vi "EnFlo_Hub.vi"() -> ()   [LabVIEW 2013]
uses:
  Anemometry Sub Vis/Controls/Launch_controls/Open_Calib.ctl
  Anemometry Sub Vis/Controls/Launch_controls/Open_Meas.ctl
  Anemometry Sub Vis/Controls/Launch_controls/Open_Enter_Temp.ctl
  Anemometry Sub Vis/Controls/Launch_controls/Multi_Run_Prog.ctl
  Anemometry Sub Vis/Controls/Launch_controls/EnFlo_arm.ctl
  Anemometry Sub Vis/Controls/Launch_controls/Fast_FID_Valve.ctl
  Anemometry Sub Vis/Controls/Launch_controls/Disp_Setup.ctl
  Anemometry Sub Vis/Controls/Launch_controls/EnFlo_Tun_Setup.ctl
  Anemometry Sub Vis/Controls/Launch_controls/User_Metadata.ctl
  Anemometry Sub Vis/Controls/Launch_controls/Trav_3D_move.ctl
  Anemometry Sub Vis/Controls/Launch_controls/Trav_Space.ctl
  Anemometry Sub Vis/Controls/Launch_controls/Tunnel_speed.ctl
  Anemometry Sub Vis/Controls/Launch_controls/Client_source_control.ctl
  Anemometry Sub Vis/Controls/Launch_controls/Hydrosonic_Manual.ctl
  Anemometry Sub Vis/Controls/Launch_controls/Preference_Panel.ctl
  Anemometry Sub Vis/Controls/Launch_controls/Hot_wire_Calculator.ctl
  Anemometry Sub Vis/Controls/Launch_controls/RW_X_Parker_Config.ctl
  Anemometry Sub Vis/Controls/Launch_controls/LDA_Alignment.ctl
  Anemometry Sub Vis/Controls/Launch_controls/Named_Serial_Comms.ctl
  Anemometry Sub Vis/Controls/Launch_controls/BSA_data_rates.ctl
  Anemometry Sub Vis/Controls/Launch_controls/Serial_Setup.ctl
  Anemometry Sub Vis/Controls/Launch_controls/Post_Process_icon.ctl
  Anemometry Sub Vis/Controls/Launch_controls/Edit_Ascii_file.ctl
  Anemometry Sub Vis/Controls/Launch_controls/Edit_Raw_DF.ctl
  Anemometry Sub Vis/Controls/Launch_controls/Results_file_plotter.ctl
  Anemometry Sub Vis/Controls/Launch_controls/Serial_Port_Names.ctl
  Anemometry Sub Vis/Controls/Launch_controls/Paul.ctl
  Anemometry Sub Vis/Controls/Launch_controls/Tom.ctl
  Anemometry Sub Vis/Controls/Launch_controls/Scani_Valve.ctl
  Anemometry Sub Vis/Controls/Launch_controls/Edit_sever_Channel.ctl
  Anemometry Sub Vis/Controls/Launch_controls/Day_file_plotter.ctl
  Anemometry Sub Vis/Controls/Launch_controls/Plot_Sever_Data.ctl
  Anemometry Sub Vis/Controls/Launch_controls/Adam_Table.ctl
  Anemometry Sub Vis/Controls/Launch_controls/Active_Channel_Control.ctl
  Anemometry Sub Vis/Controls/Setup.ctl
  Anemometry Sub Vis/Controls/Post_Process.ctl
  Anemometry Sub Vis/Controls/Preference_Mode.ctl
  Anemometry Sub Vis/Gen Trav/Trav_mode.ctl
  Anemometry Sub Vis/Controls/User_Specific_mode.ctl
  Anemometry Sub Vis/File/Setup_Filetype.ctl
  Anemometry Sub Vis/Calibration/Calib_mode.ctl
  Anemometry Sub Vis/Controls/Server_Comms.ctl
  Anemometry Sub Vis/Controls/App_Global.ctl
  Anemometry Sub Vis/Globals/Dynamic_call_global.ph.vi
  Anemometry Sub Vis/Globals/Constants_global.vi
  Anemometry Sub Vis/Globals/Preference_global.vi
  Anemometry Sub Vis/Globals/Meas_global.vi
  <vilib>/Platform/browser.llb/Open URL in Default Browser (string).vi
  Anemometry Sub Vis/Globals/Trav_pos_global.vi
  Anemometry Sub Vis/Acquisition/PWA/PWAtasksGLOBAL.vi
  Anemometry Sub Vis/Utilities/Email_transfer_global.vi
panel:
  out "List of ADAM channels to view":string[](array[string])
  out "List of ADAM control channels":string[](array[string])
  out "Analogue Dev Name":string="Dev2"
  out "Numeric":i32
  out "Rig Name":string="EnFlo Tunnel"
  out "All Users":path=path "/System Folder/Preferences/LabVIEW (EnFlo specific)/Meas Setups"
  out "Dummy Measurement":bool
  in  "stop":bool
  in  "Tab Control":T1(tab)
  in  "Tunnel Speed Control":T2
  in  "Traverse Space":T3
  in  "Trav 3D Move":T4 caption="3D Traverse Move"
  in  "User Metadata":T5
  in  "Multi Run Prog":T6
  in  "Enter Temp_Press":T7
  in  "Measurement Prog":T8 caption="Measurement"
  in  "Calibration Prog":T9 caption="Calibration"
  in  "Scani Valve":T10
  in  "LDA Alignment":T11
  in  "Hydrosonic Control":T12
  in  "Fast FID Valve":T13
  in  "Source Control":T14
  in  "Gas Release Setup":T15
  in  "EnFlo Tunnel Setup":T16
  in  "Heater Setup":bool caption="Inlet heater File"
  in  "EnFlo Arm":T17
  in  "EnFlo Tun Display":bool
  in  "Rig_Control":cluster{"Ch Name":string, "Boolean":bool}[](array[cluster])
  in  "ADAM Channels Control":T18 caption="Change Active Channels"
  in  "ADAM Scan Table":T19 caption="Run ADAM Scan Table"
  in  "Edit Server Channel":T20
  in  "Plot Server Channels":T21 caption="Plot Server Data"
  in  "Day Files Plotter":T22 caption="Plot Data From File"
  out "Current Values":cluster{"Ch Name":string, "Numeric":dbl}[](array[cluster])
  in  "Post_Pro_Results_Hierarchy":bool
  in  "Results File Plotter":T23
  in  "Edit Raw Data Files":T24
  in  "Edit ASCII File":T25
  in  "Post Process Raw Data":T26
  in  "Top Level Traverse":bool
  in  "Show Manual Sync":bool
  in  "Sync to server now":bool
  in  "Port Names":T27
  in  "Serial Setup":T28
  in  "LDA Data Rate":T29
  in  "Named Serial Comms":T30
  in  "RW Trav Setup":T31
  in  "Hot Wire Calc":T32
  in  "Preference Panel":T33
  in  "Tom Lawton t.lawton@surrey.ac.uk":T34 caption="For hardware support"
  in  "Paul Hayden p.hayden@surrey.ac.uk":T35 caption="For software support"
  in  "Online Manual":bool
  out "VI Name":string
  out "Iterations":i32
  # "Or give us a call on Tel: 01483 689545"
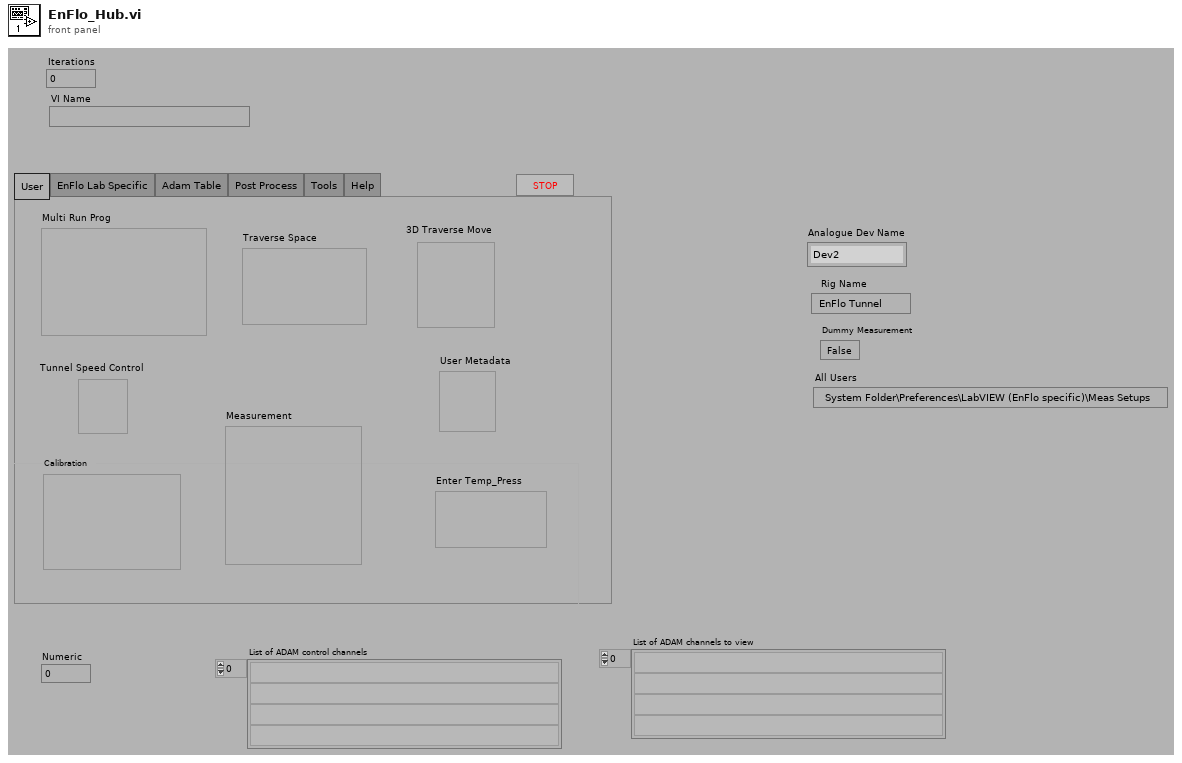
[diagram p1: front panel]
types:
  T1 = enum32{"User", "EnFlo Lab Specific", "Adam Table", "Post Process", "Tools", "Help"}
  T2 = typedef "Tunnel_speed.ctl" = bool
  T3 = typedef "Trav_Space.ctl" = bool
  T4 = typedef "Trav_3D_move.ctl" = bool
  T5 = typedef "User_Metadata.ctl" = bool
  T6 = typedef "Multi_Run_Prog.ctl" = bool
  T7 = typedef "Open_Enter_Temp.ctl" = bool
  T8 = typedef "Open_Meas.ctl" = bool
  T9 = typedef "Open_Calib.ctl" = bool
  T10 = typedef "Scani_Valve.ctl" = bool
  T11 = typedef "LDA_Alignment.ctl" = bool
  T12 = typedef "Hydrosonic_Manual.ctl" = bool
  T13 = typedef "Fast_FID_Valve.ctl" = bool
  T14 = typedef "Client_source_control.ctl" = bool
  T15 = typedef "Disp_Setup.ctl" = bool
  T16 = typedef "EnFlo_Tun_Setup.ctl" = bool
  T17 = typedef "EnFlo_arm.ctl" = bool
  T18 = typedef "Active_Channel_Control.ctl" = bool
  T19 = typedef "Adam_Table.ctl" = bool
  T20 = typedef "Edit_sever_Channel.ctl" = bool
  T21 = typedef "Plot_Sever_Data.ctl" = bool
  T22 = typedef "Day_file_plotter.ctl" = bool
  T23 = typedef "Results_file_plotter.ctl" = bool
  T24 = typedef "Edit_Raw_DF.ctl" = bool
  T25 = typedef "Edit_Ascii_file.ctl" = bool
  T26 = typedef "Post_Process_icon.ctl" = bool
  T27 = typedef "Serial_Port_Names.ctl" = bool
  T28 = typedef "Serial_Setup.ctl" = bool
  T29 = typedef "BSA_data_rates.ctl" = bool
  T30 = typedef "Named_Serial_Comms.ctl" = bool
  T31 = typedef "RW_X_Parker_Config.ctl" = bool
  T32 = typedef "Hot_wire_Calculator.ctl" = bool
  T33 = typedef "Preference_Panel.ctl" = bool
  T34 = typedef "Tom.ctl" = bool
  T35 = typedef "Paul.ctl" = bool
  T36 = enum32{"invalid app kind", "Development System", "Run Time System", "Student Edition", "Embedded LabVIEW", "Evaluation", "Custom"}
  T37 = typedef "Post_Process.ctl" = enum16{"Take New Data", "Post Process Raw Data File"}
  T38 = typedef "Setup.ctl" = enum16{"Run Program", "Show Setup", "Save Current Setup", "Setup Front Panel"}
  T39 = enum16{"Get Channel Names", "Get Current Value", "Update Channel Value", "Update Channel Description"}
  T40 = enum32{"Invalid", "Standard", "Closed", "Hidden", "Minimized", "Maximized"}
  T41 = typedef "Preference_Mode.ctl" = enum16{"Load Preferences from file", "Save Preferences to file", "Load, Edit then Save"}
  T42 = typedef "User_Specific_mode.ctl" = enum16{"Check VI only", "Run VI"}
  T43 = typedef "Trav_mode.ctl" = enum16{"Move traverse", "Read traverse position", "Teach Position"}
  T44 = typedef "Setup_Filetype.ctl" = enum16{"Measurement Setups", "Calibration Setups", "General", "Results File Plotter Setups", "Speed Calib Tweaks"}
  T45 = enum16{"Load Command File", "Save Command File", "Check Multi Run Prog", "Check Multi Run Prog With Live Moves", "Run Multi Run Prog"}
  T46 = typedef "Calib_mode.ctl" = enum16{"Show Setup", "Take a New Calibration Point", "Refit Curve", "Setup Front Panel"}
  T47 = typedef "Tunnel_Coordinates.ctl" = enum16{"Work in Tunnel Coordinates", "Work in Model Coordinates"}
  T48 = typedef "App_Global.ctl" = enum16{"Read Global", "Write to Global", "Initialise Array"}
  T49 = typedef "App_Ref_Cluster.ctl" = cluster{"Server IP & Port No":string, "Application reference":refnum<vi>}
  T50 = typedef "Server_Comms.ctl" = enum16{"Server Link Healthy", "Do Not Link To Server"}
  T51 = typedef "Ch_description_ADAM.ctl" = cluster{"Ch Name":string, "Type":T52, "Function":T53, "Ch State":T54, "Calibration type":T55, "A":dbl, "B":dbl, "C":dbl, "D":dbl, "Comments":string, "Address":T56, "String":string, "Duty":u16}
  T52 = typedef "Module_type_ADAM.ctl" = string
  T53 = typedef "Function_ADAM.ctl" = enum16{"Analogue Input", "Digital Input", "Event counter", "Event rate", "Analogue Output", "Digital Output", "Relay Output"}
  T54 = typedef "Channel_State.ctl" = enum16{"On", "Off", "Always On", "Always Off"}
  T55 = typedef "Calib_type_ADAM.ctl" = enum16{"Raw", "Bx + A", "Cx^2 + Bx + A", "Dx^3 + Cx^2 + Bx + A", "In Band", "Hi-Tec Q", "Hi-Tec M_dot", "Text"}
  T56 = typedef "Address.ctl" = cluster{"Main":i32, "Ch.":i32, "Sub":i32, "Port Name":string}
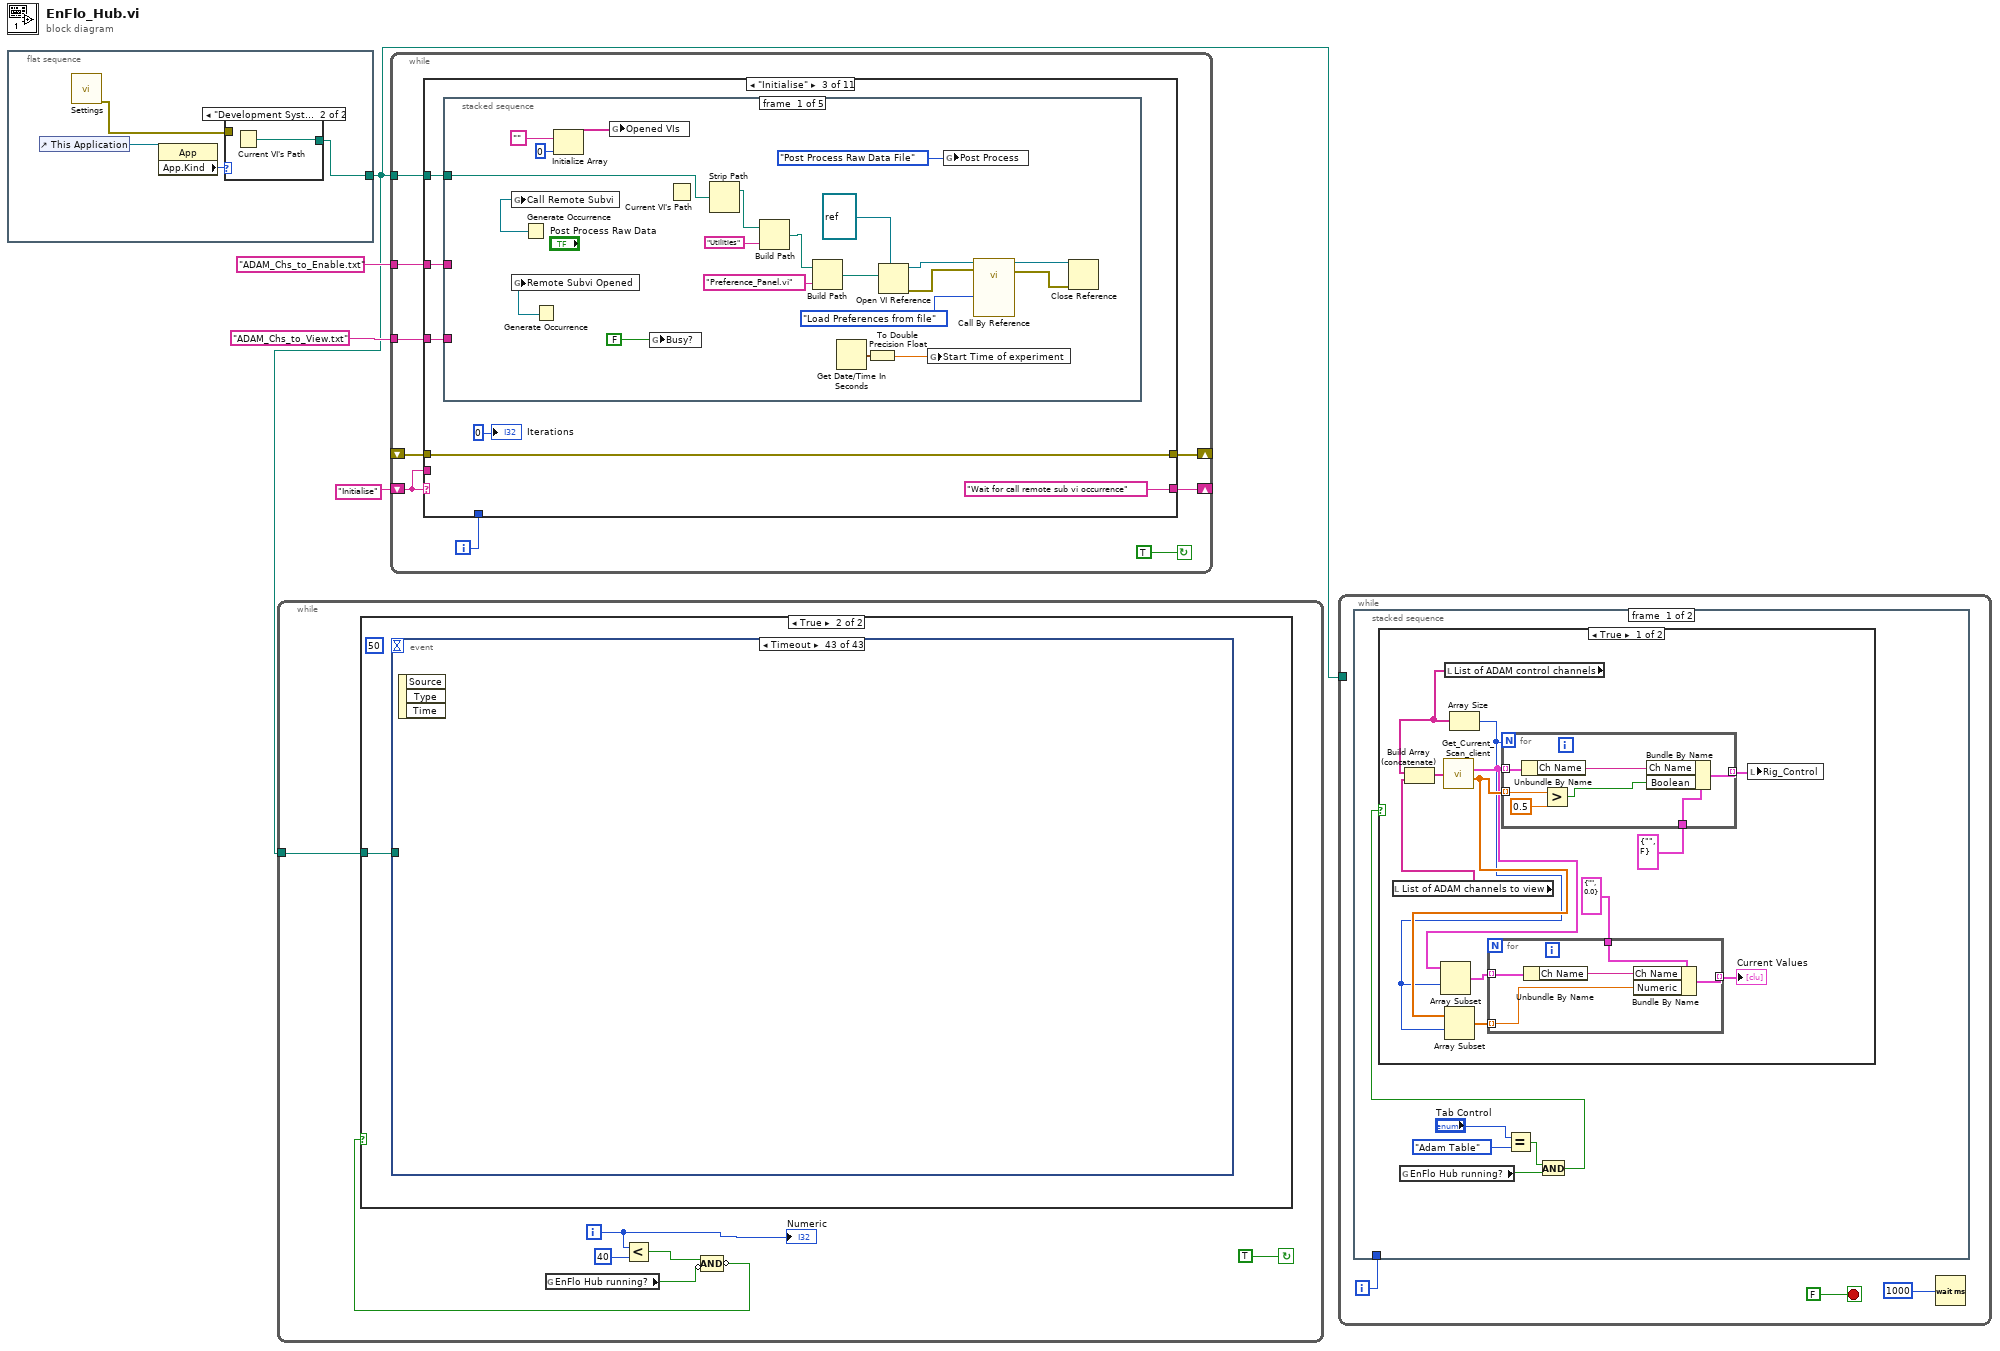
[diagram p0: block diagram]
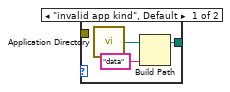
[diagram p2: hidden frame]
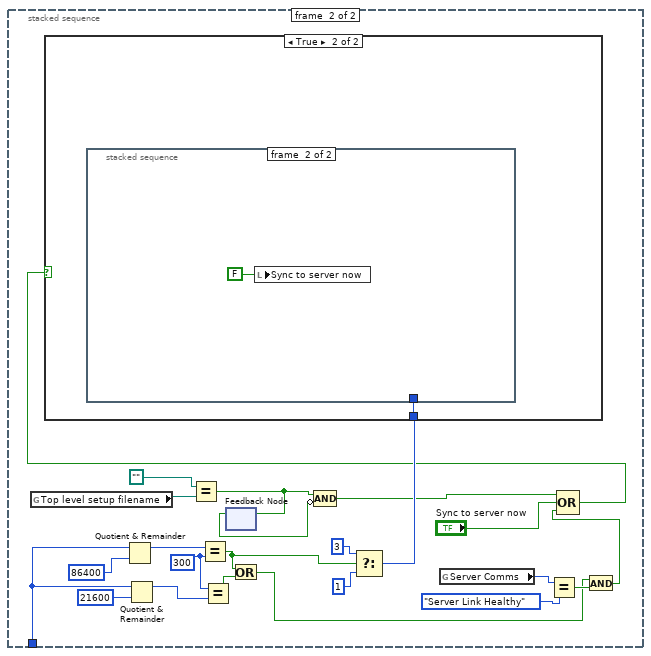
[diagram p4: hidden frame]
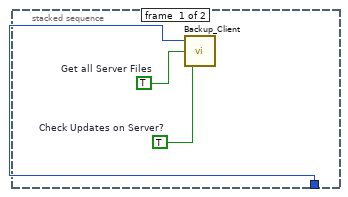
[diagram p6: hidden frame]
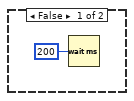
[diagram p7: hidden frame]
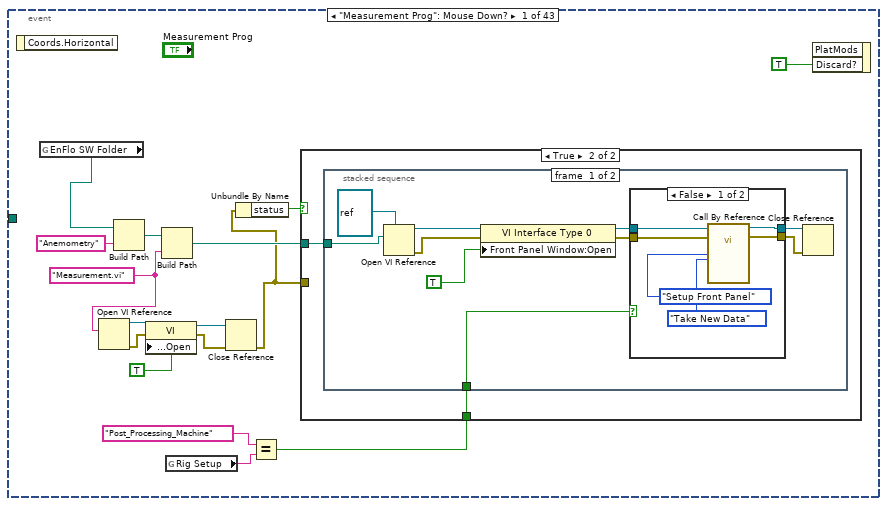
[diagram p8: hidden frame]
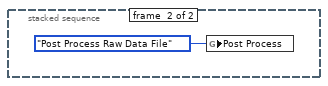
[diagram p11: hidden frame]
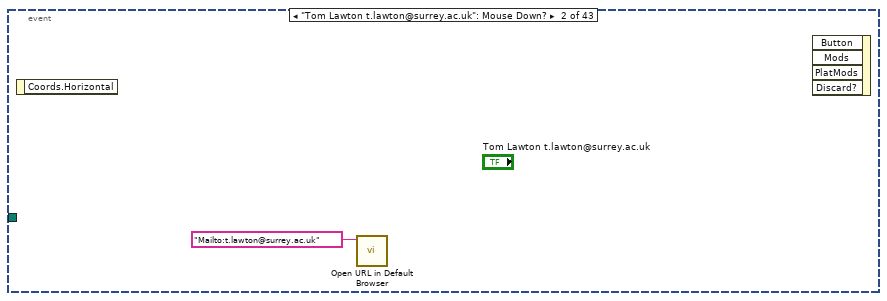
[diagram p12: hidden frame]
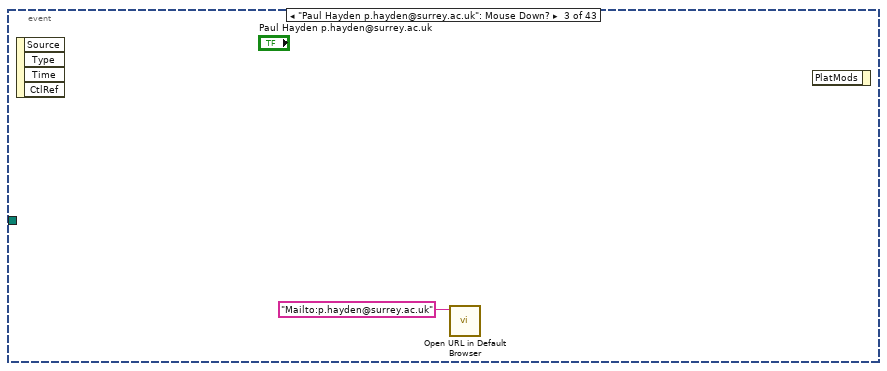
[diagram p13: hidden frame]
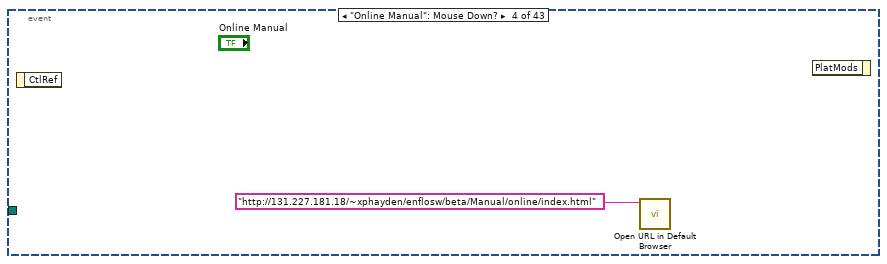
[diagram p14: hidden frame]
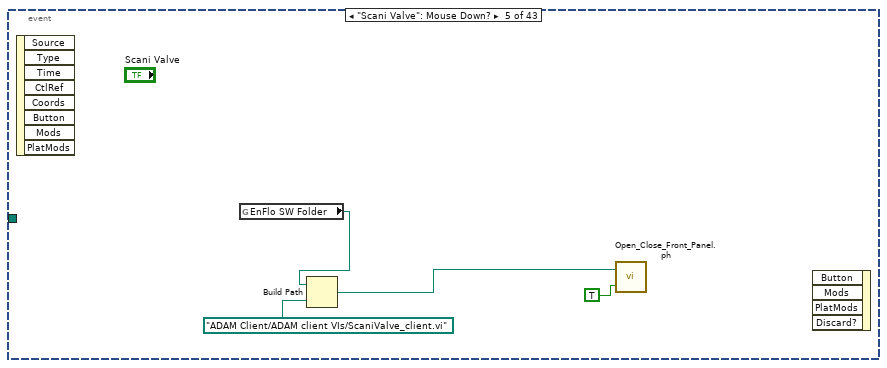
[diagram p15: hidden frame]
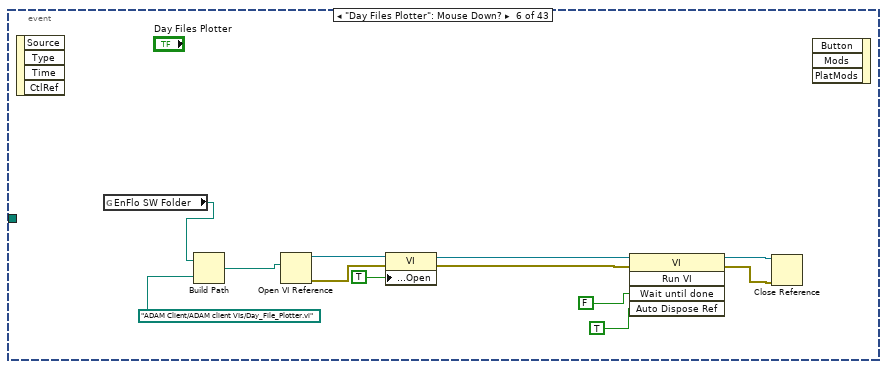
[diagram p16: hidden frame]
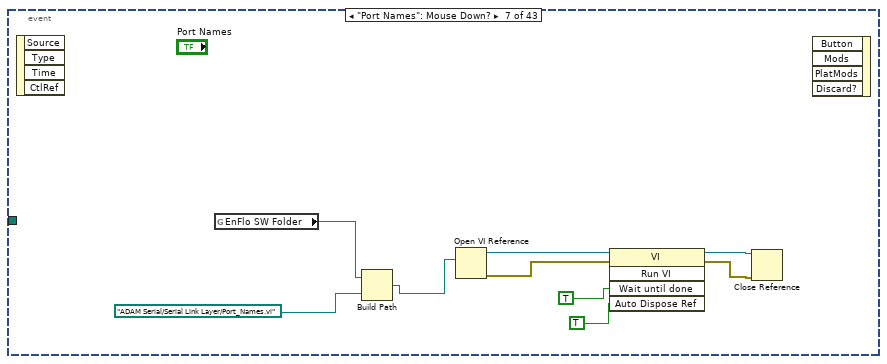
[diagram p17: hidden frame]
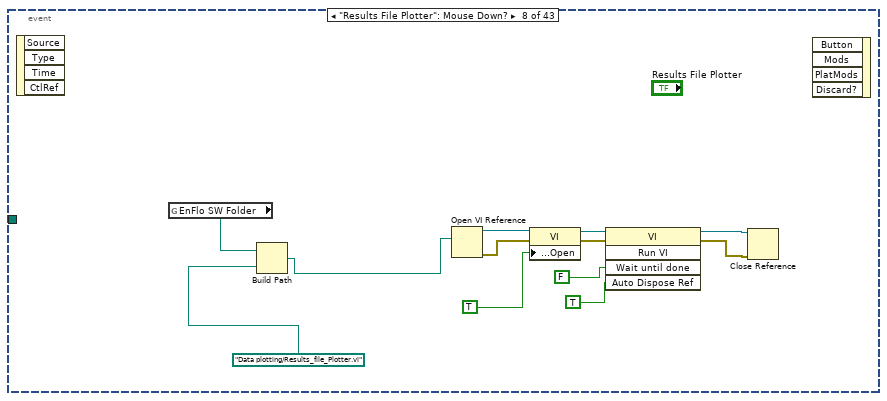
[diagram p18: hidden frame]
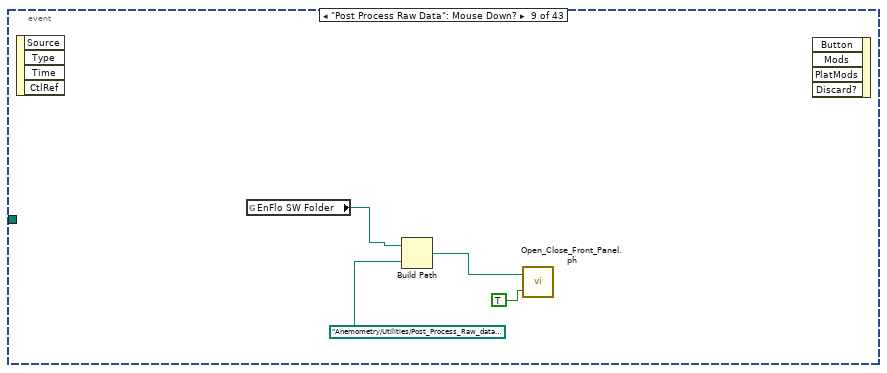
[diagram p19: hidden frame]
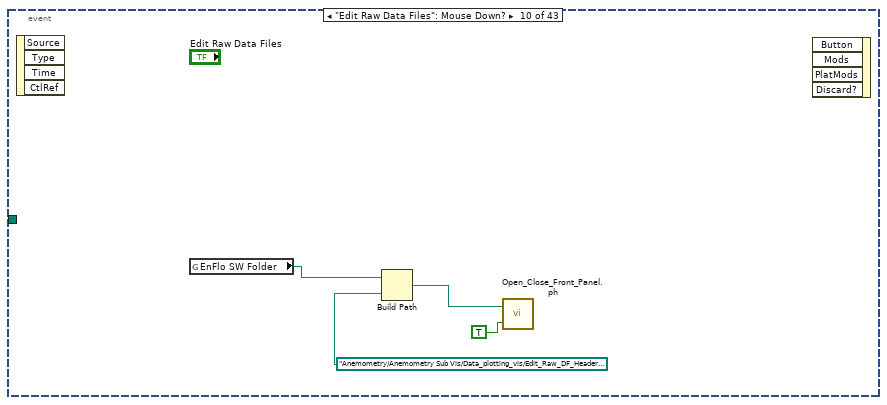
[diagram p20: hidden frame]
diagram:
  n1 = flat-sequence {
    tunnel: [w8] -> w1
    frame #0 {
      n2 = control-ref of="This Application"() -> (w6:refnum<vi>)
      n3 = call "Settings.vi"() -> ("error out"=w5:errorcluster)  [unwired: 11 in]
      n4 = property class="App"(reference=w6) -> ("App.Kind"=w7:T36)  [unwired: 1 in, 2 out]
      n5 = case shown="\"Development System\"" w7 {
        tunnel: [w11 w12] -> w8
        tunnel: w5 -> [_ _]
        frame "invalid app kind", Default {
          n6 = call <vilib>:"Application Directory.vi"() -> ("Application Directory"=w9:path)
          n7 = Build Path(base path=w9, name or relative path="data") -> (appended path=w11:path)
        }
        frame "Development System" {
          n8 = Current VI's Path() -> (path=w12:path)
        }
      }
    }
  }
  n9 = while {
    tunnel: w1 -> [w13]
    i -> [w18]
    stop <- TRUE continue-if-true
    n10 = global read "Dynamic_call_global.ph.vi" "EnFlo Hub running?"() -> (w16:bool)
    n11 = Less?(x=w18, y=40) -> (x < y?=w15:bool)
    n12 = Compound Arithmetic op=AND(w15, invert w16) -> (invert w14:bool)
    n13 = case shown="True" w14 {
      tunnel: w13 -> [_ w21]
      frame False {
        n14 = Wait (ms)(milliseconds to wait=u32 200) -> ()  [unwired: 1 out]
      }
      frame True {
        (unwired) 50
        n15 = event shown="[42] Timeout" {
          selector: _ -> [_ _ _ _ _ _ _ _ _ _ _ _ _ _ _ _ _ _ _ _ _ _ _ _ _ _ _ _ _ _ _ _ _ _ _ _ _ _ _ _ _ _ _]
          dyn-events: _ -> [_ _ _ _ _ _ _ _ _ _ _ _ _ _ _ _ _ _ _ _ _ _ _ _ _ _ _ _ _ _ _ _ _ _ _ _ _ _ _ _ _ _ _]
          timeout: _ -> [_ _ _ _ _ _ _ _ _ _ _ _ _ _ _ _ _ _ _ _ _ _ _ _ _ _ _ _ _ _ _ _ _ _ _ _ _ _ _ _ _ _ _]
          tunnel: w21 -> [_ _ _ _ _ _ _ _ _ _ _ _ _ _ _ _ _ _ _ _ _ _ _ _ _ _ _ _ _ _ _ _ _ _ _ _ _ _ _ _ _ _ _]
          event "Measurement Prog": Mouse Down? {
            w30 = "Measurement.vi" ("name or relative path")
            n16 = event-data() -> ()  [unwired: 2 out]
            n17 = global read "Constants_global.vi" "EnFlo SW Folder"() -> (w33:path)
            n18 = Open VI Reference(vi path=w30) -> (vi reference=w29:refnum<vi>, error out=w28:errorcluster)  [unwired: 1 in, 4 out]
            n19 = Build Path(base path=w33, name or relative path="Anemometry") -> (appended path=w36:path)
            n20 = property class="VI"(reference=w29, error in=w28, "Front Panel Window:Open"=TRUE) -> (reference out=w26:refnum<vi>, error out=w27:errorcluster)
            n21 = Build Path(base path=w36, name or relative path=w30) -> (appended path=w34:path)
            n22 = global read "Preference_global.vi" "Rig Setup"() -> (w24:string)
            n23 = Close Reference(reference=w26, error in (no error)=w27) -> (error out=w25:errorcluster)
            n24 = Unbundle By Name(w25) -> ("status"=w35:bool)
            n25 = Equal?(x="Post_Processing_Machine" ("Rig Setup"), y=w24) -> (x = y?=w22:bool)
            n26 = case shown="True" w35 {
              tunnel: w34 -> [_ w39]
              tunnel: w25 -> [_ _]
              tunnel: w22 -> [_ w38]
              frame False {
              }
              frame True {
                n27 = stacked-sequence {
                  tunnel: w39 -> [w49 _]
                  tunnel: w38 -> [w40 _]
                  frame #0 {
                    n28 = Open VI Reference(type specifier VI Refnum (for type only)=refnum<vi> refnum, vi path=w49) -> (vi reference=w47:refnum<vi>, error out=w46:errorcluster)  [unwired: 1 in, 3 out]
                    n29 = property class="VI Interface Type 0"(reference=w47, error in=w46, "Front Panel Window:Open"=TRUE) -> (reference out=w42:refnum<vi>, error out=w41:errorcluster)
                    n30 = case shown="False" w40 {
                      tunnel: [w55 w57] -> w45
                      tunnel: [w54 w56] -> w44
                      tunnel: w42 -> [w53 w57]
                      tunnel: w41 -> [w52 w56]
                      frame False {
                        n31 = call-by-ref "?"(reference=w53, error in=w52, "setup"=Setup."Setup Front Panel", "Post Process"=Post_Process."Take New Data") -> (reference out=w55:refnum<vi>, error out=w54:errorcluster)  [unwired: 16 in, 2 out]
                      }
                      frame True {
                      }
                    }
                    n32 = Close Reference(reference=w45, error in (no error)=w44) -> ()  [unwired: 1 out]
                  }
                  frame #1 {
                    n33 = global write "Meas_global.vi" "Post Process"(Post_Process."Post Process Raw Data File" ("Post Process")) -> ()
                  }
                }
              }
            }
            n34 = event-data("Discard?"=TRUE) -> ()  [unwired: 1 in, 2 out]
          }
          event "Tom Lawton t.lawton@surrey.ac.uk": Mouse Down? {
            n35 = event-data() -> ()  [unwired: 2 out]
            n36 = call-poly <vilib>:"Open URL in Default Browser.vi"("URL"="Mailto:t.lawton@surrey.ac.uk") -> ()  [unwired: 1 in, 6 out]
            n37 = event-data() -> ()  [unwired: 1 in, 5 out]
          }
          event "Paul Hayden p.hayden@surrey.ac.uk": Mouse Down? {
            n38 = event-data() -> ()  [unwired: 5 out]
            n39 = call-poly <vilib>:"Open URL in Default Browser.vi"("URL"="Mailto:p.hayden@surrey.ac.uk") -> ()  [unwired: 1 in, 6 out]
            n40 = event-data() -> ()  [unwired: 1 in, 2 out]
          }
          event "Online Manual": Mouse Down? {
            n41 = event-data() -> ()  [unwired: 2 out]
            n42 = call-poly <vilib>:"Open URL in Default Browser.vi"("URL"="http://131.227.181.18/~xphayden/enflosw/beta/Manual/online/index.html") -> ()  [unwired: 1 in, 6 out]
            n43 = event-data() -> ()  [unwired: 1 in, 2 out]
          }
          event "Scani Valve": Mouse Down? {
            n44 = event-data() -> ()  [unwired: 9 out]
            n45 = global read "Constants_global.vi" "EnFlo SW Folder"() -> (w62:path)
            n46 = Build Path(base path=w62, name or relative path=path "ADAM Client/ADAM client VIs/ScaniValve_client.vi") -> (appended path=w65:path)
            n47 = call "Open_Close_Front_Panel.ph.vi"("Front Panel Window:Open"=TRUE, "VI path"=w65) -> ()  [unwired: 2 out]
            n48 = event-data() -> ()  [unwired: 1 in, 5 out]
          }
          event "Day Files Plotter": Mouse Down? {
            n49 = event-data() -> ()  [unwired: 5 out]
            n50 = global read "Constants_global.vi" "EnFlo SW Folder"() -> (w66:path)
            n51 = Build Path(base path=w66, name or relative path=path "ADAM Client/ADAM client VIs/Day_File_Plotter.vi") -> (appended path=w72:path)
            n52 = Open VI Reference(vi path=w72) -> (vi reference=w73:refnum<vi>, error out=w75:errorcluster)  [unwired: 2 in, 3 out]
            n53 = property class="VI"(reference=w73, error in=w75, "Front Panel Window:Open"=TRUE) -> (reference out=w77:refnum<vi>, error out=w76:errorcluster)
            n54 = invoke class="VI" method="Run VI"(reference=w77, error in=w76, "Wait until done"=FALSE, "Auto Dispose Ref"=TRUE) -> (reference out=w68:refnum<vi>, error out=w69:errorcluster)  [unwired: 1 in, 3 out]
            n55 = Close Reference(reference=w68, error in (no error)=w69) -> ()  [unwired: 1 out]
            n56 = event-data() -> ()  [unwired: 1 in, 4 out]
          }
          event "Port Names": Mouse Down? {
            n57 = event-data() -> ()  [unwired: 5 out]
            n58 = global read "Constants_global.vi" "EnFlo SW Folder"() -> (w78:path)
            n59 = Build Path(base path=w78, name or relative path=path "ADAM Serial/Serial Link Layer/Port_Names.vi") -> (appended path=w80:path)
            n60 = Open VI Reference(vi path=w80) -> (vi reference=w85:refnum<vi>, error out=w86:errorcluster)  [unwired: 1 in, 4 out]
            n61 = invoke class="VI" method="Run VI"(reference=w85, error in=w86, "Wait until done"=TRUE, "Auto Dispose Ref"=TRUE) -> (reference out=w81:refnum<vi>, error out=w82:errorcluster)  [unwired: 1 in, 3 out]
            n62 = Close Reference(reference=w81, error in (no error)=w82) -> ()  [unwired: 1 out]
            n63 = event-data() -> ()  [unwired: 1 in, 5 out]
          }
          event "Results File Plotter": Mouse Down? {
            n64 = event-data() -> ()  [unwired: 5 out]
            n65 = global read "Constants_global.vi" "EnFlo SW Folder"() -> (w87:path)
            n66 = Build Path(base path=w87, name or relative path=path "Data plotting/Results_file_Plotter.vi") -> (appended path=w90:path)
            n67 = Open VI Reference(vi path=w90) -> (vi reference=w92:refnum<vi>, error out=w89:errorcluster)  [unwired: 1 in, 4 out]
            n68 = property class="VI"(reference=w92, error in=w89, "Front Panel Window:Open"=TRUE) -> (reference out=w93:refnum<vi>, error out=w94:errorcluster)
            n69 = invoke class="VI" method="Run VI"(reference=w93, error in=w94, "Wait until done"=FALSE, "Auto Dispose Ref"=TRUE) -> (reference out=w95:refnum<vi>, error out=w96:errorcluster)  [unwired: 1 in, 3 out]
            n70 = Close Reference(reference=w95, error in (no error)=w96) -> ()  [unwired: 1 out]
            n71 = event-data() -> ()  [unwired: 1 in, 5 out]
          }
          event "Post Process Raw Data": Mouse Down? {
            n72 = event-data() -> ()  [unwired: 5 out]
            n73 = global read "Constants_global.vi" "EnFlo SW Folder"() -> (w99:path)
            n74 = Build Path(base path=w99, name or relative path=path "Anemometry/Utilities/Post_Process_Raw_data.vi") -> (appended path=w101:path)
            n75 = call "Open_Close_Front_Panel.ph.vi"("Front Panel Window:Open"=TRUE, "VI path"=w101) -> ()  [unwired: 2 out]
            n76 = event-data() -> ()  [unwired: 1 in, 5 out]
          }
          event "Edit Raw Data Files": Mouse Down? {
            n77 = event-data() -> ()  [unwired: 5 out]
            n78 = global read "Constants_global.vi" "EnFlo SW Folder"() -> (w103:path)
            n79 = Build Path(base path=w103, name or relative path=path "Anemometry/Anemometry Sub Vis/Data_plotting_vis/Edit_Raw_DF_Header.vi") -> (appended path=w105:path)
            n80 = call "Open_Close_Front_Panel.ph.vi"("Front Panel Window:Open"=TRUE, "VI path"=w105) -> ()  [unwired: 2 out]
            n81 = event-data() -> ()  [unwired: 1 in, 5 out]
          }
          event "Serial Setup": Mouse Down? {
            n82 = event-data() -> ()  [unwired: 5 out]
            n83 = global read "Constants_global.vi" "EnFlo SW Folder"() -> (w107:path)
            n84 = Build Path(base path=w107, name or relative path=path "ADAM Serial/Serial Link Layer/Serial_Setup.vi") -> (appended path=w109:path)
            n85 = Open VI Reference(vi path=w109) -> (vi reference=w114:refnum<vi>, error out=w115:errorcluster)  [unwired: 1 in, 4 out]
            n86 = invoke class="VI" method="Run VI"(reference=w114, error in=w115, "Wait until done"=TRUE, "Auto Dispose Ref"=TRUE) -> (reference out=w110:refnum<vi>, error out=w111:errorcluster)  [unwired: 1 in, 3 out]
            n87 = Close Reference(reference=w110, error in (no error)=w111) -> ()  [unwired: 1 out]
            n88 = event-data() -> ()  [unwired: 1 in, 2 out]
          }
          event "Named Serial Comms": Mouse Down? {
            n89 = event-data() -> ()  [unwired: 5 out]
            n90 = global read "Constants_global.vi" "EnFlo SW Folder"() -> (w117:path)
            n91 = Build Path(base path=w117, name or relative path=path "ADAM Serial/Serial Link Layer/Named_Serial_Comms.vi") -> (appended path=w119:path)
            n92 = call "Open_Close_Front_Panel.ph.vi"("Front Panel Window:Open"=TRUE, "VI path"=w119) -> ()  [unwired: 2 out]
            n93 = event-data() -> ()  [unwired: 1 in, 5 out]
          }
          event "LDA Data Rate": Mouse Down? {
            n94 = event-data() -> ()  [unwired: 5 out]
            n95 = global read "Constants_global.vi" "EnFlo SW Folder"() -> (w120:path)
            n96 = Build Path(base path=w120, name or relative path=path "Anemometry/Anemometry Sub Vis/LDA/LDA_data_rate.vi") -> (appended path=w122:path)
            n97 = call "Open_Close_Front_Panel.ph.vi"("Front Panel Window:Open"=TRUE, "VI path"=w122) -> ()  [unwired: 2 out]
            n98 = event-data() -> ()  [unwired: 1 in, 2 out]
          }
          event "ADAM Channels Control": Mouse Down? {
            n99 = event-data() -> ()  [unwired: 5 out]
            n100 = global read "Constants_global.vi" "EnFlo SW Folder"() -> (w134:path)
            n101 = Build Path(base path=w134, name or relative path=path "ADAM Client/ADAM client VIs/Control_Channel_Status.vi") -> (appended path=w124:path)
            n102 = Open VI Reference(vi path=w124) -> (vi reference=w127:refnum<vi>, error out=w125:errorcluster)  [unwired: 1 in, 4 out]
            n103 = property class="VI"(reference=w127, error in=w125, "Front Panel Window:Open"=TRUE) -> (reference out=w128:refnum<vi>, error out=w129:errorcluster)
            n104 = invoke class="VI" method="Run VI"(reference=w128, error in=w129, "Wait until done"=FALSE, "Auto Dispose Ref"=TRUE) -> (reference out=w130:refnum<vi>, error out=w131:errorcluster)  [unwired: 1 in, 3 out]
            n105 = Close Reference(reference=w130, error in (no error)=w131) -> ()  [unwired: 1 out]
            n106 = event-data() -> ()  [unwired: 1 in, 2 out]
          }
          event "LDA Alignment": Mouse Down? {
            n107 = event-data() -> ()  [unwired: 5 out]
            n108 = global read "Constants_global.vi" "EnFlo SW Folder"() -> (w136:path)
            n109 = Build Path(base path=w136, name or relative path=path "Anemometry/Utilities/LDA_Beam_Alignment.vi") -> (appended path=w138:path)
            n110 = call "Open_Close_Front_Panel.ph.vi"("Front Panel Window:Open"=TRUE, "VI path"=w138) -> ()  [unwired: 2 out]
            n111 = event-data() -> ()  [unwired: 1 in, 5 out]
          }
          event "Enter Temp_Press": Mouse Down? {
            w141 = FALSE  # Wait until done
            n112 = event-data() -> ()  [unwired: 5 out]
            n113 = call "Run_Enter_Temp.vi"("Wait until done"=w141) -> ()  [unwired: 1 out]
            n114 = event-data("Discard?"=TRUE) -> ()  [unwired: 1 in, 4 out]
          }
          event "Edit ASCII File": Mouse Down? {
            n115 = event-data() -> ()  [unwired: 5 out]
            n116 = global read "Constants_global.vi" "EnFlo SW Folder"() -> (w142:path)
            n117 = Build Path(base path=w142, name or relative path=path "Anemometry/Utilities/Edit_ASCI_file.vi") -> (appended path=w145:path)
            n118 = call "Open_Close_Front_Panel.ph.vi"("Front Panel Window:Open"=TRUE, "VI path"=w145) -> ()  [unwired: 2 out]
            n119 = event-data() -> ()  [unwired: 1 in, 5 out]
          }
          event "Heater Setup": Mouse Down? {
            n120 = event-data() -> ()  [unwired: 5 out]
            n121 = global read "Constants_global.vi" "EnFlo SW Folder"() -> (w146:path)
            n122 = Build Path(base path=w146, name or relative path=path "Anemometry/Utilities/Create_Heater_Setpoints_File.vi") -> (appended path=w149:path)
            n123 = call "Open_Close_Front_Panel.ph.vi"("Front Panel Window:Open"=TRUE, "VI path"=w149) -> ()  [unwired: 2 out]
            n124 = event-data() -> ()  [unwired: 1 in, 5 out]
          }
          event "Source Control": Mouse Down? {
            n125 = event-data() -> ()  [unwired: 5 out]
            n126 = global read "Constants_global.vi" "EnFlo SW Folder"() -> (w150:path)
            n127 = Build Path(base path=w150, name or relative path=path "ADAM Client/Sub VIs/Gas_Release_Control.vi") -> (appended path=w153:path)
            n128 = call "Open_Close_Front_Panel.ph.vi"("Front Panel Window:Open"=TRUE, "VI path"=w153) -> ()  [unwired: 2 out]
            n129 = event-data() -> ()  [unwired: 1 in, 5 out]
          }
          event "Edit Server Channel": Mouse Down? {
            n130 = event-data() -> ()  [unwired: 5 out]
            n131 = global read "Constants_global.vi" "EnFlo SW Folder"() -> (w154:path)
            n132 = Build Path(base path=w154, name or relative path=path "ADAM Client/ADAM client VIs/Edit_Server_Channel.vi") -> (appended path=w164:path)
            n133 = Open VI Reference(type specifier VI Refnum (for type only)=refnum<vi> refnum, vi path=w164) -> (vi reference=w157:refnum<vi>, error out=w158:errorcluster)  [unwired: 1 in, 3 out]
            n134 = property class="VI Interface Type 1"(reference=w157, error in=w158, "Front Panel Window:Open"=TRUE) -> (reference out=w160:refnum<vi>, error out=w161:errorcluster)
            n135 = call-by-ref "?"(reference=w160, error in=w161, "Mode"=T39."Get Channel Names") -> (reference out=w162:refnum<vi>, error out=w163:errorcluster)  [unwired: 5 in]
            n136 = Close Reference(reference=w162, error in (no error)=w163) -> ()  [unwired: 1 out]
            n137 = event-data() -> ()  [unwired: 1 in, 5 out]
          }
          event "EnFlo Tun Display": Mouse Down? {
            n138 = event-data() -> ()  [unwired: 9 out]
            n139 = global read "Constants_global.vi" "EnFlo SW Folder"() -> (w177:path)
            n140 = Build Path(base path=w177, name or relative path=path "Anemometry/Utilities/EnFlo_Tunnel_Display.vi") -> (appended path=w172:path)
            n141 = Open VI Reference(vi path=w172) -> (vi reference=w171:refnum<vi>, error out=w170:errorcluster)  [unwired: 5 in]
            n142 = invoke class="VI" method="FP.Open"(reference=w171, error in=w170, "Activate"=TRUE ("Activate?"), "State"=T40."Standard") -> (reference out=w169:refnum<vi>, error out=w168:errorcluster)  [unwired: 1 in, 3 out]
            n143 = invoke class="VI" method="Run VI"(reference=w169, error in=w168, "Wait until done"=FALSE ("Wait Until Done"), "Auto Dispose Ref"=FALSE ("Wait until done")) -> (reference out=w173:refnum<vi>, error out=w174:errorcluster)  [unwired: 1 in, 3 out]
            n144 = Close Reference(reference=w173, error in (no error)=w174) -> ()  [unwired: 1 out]
            n145 = event-data() -> ()  [unwired: 5 in, 1 out]
          }
          event "Tunnel Speed Control": Mouse Down? {
            n146 = event-data() -> ()  [unwired: 5 out]
            n147 = global read "Constants_global.vi" "EnFlo SW Folder"() -> (w179:path)
            n148 = Build Path(base path=w179, name or relative path=path "ADAM Client/ADAM client VIs/Set_Tunnel_Speed.vi") -> (appended path=w182:path)
            n149 = call "Open_Close_Front_Panel.ph.vi"("Front Panel Window:Open"=TRUE, "VI path"=w182) -> ()  [unwired: 2 out]
            n150 = event-data() -> ()  [unwired: 1 in, 5 out]
          }
          event "Plot Server Channels": Mouse Down? {
            n151 = event-data() -> ()  [unwired: 5 out]
            n152 = global read "Constants_global.vi" "EnFlo SW Folder"() -> (w183:path)
            n153 = Build Path(base path=w183, name or relative path=path "ADAM Client/ADAM client VIs/Plot_Server_Data.vi") -> (appended path=w186:path)
            n154 = Open VI Reference(vi path=w186) -> (vi reference=w188:refnum<vi>, error out=w185:errorcluster)  [unwired: 1 in, 4 out]
            n155 = property class="VI"(reference=w188, error in=w185, "Front Panel Window:Open"=TRUE) -> (reference out=w189:refnum<vi>, error out=w190:errorcluster)
            n156 = invoke class="VI" method="Run VI"(reference=w189, error in=w190, "Wait until done"=FALSE, "Auto Dispose Ref"=TRUE) -> (reference out=w191:refnum<vi>, error out=w192:errorcluster)  [unwired: 1 in, 3 out]
            n157 = Close Reference(reference=w191, error in (no error)=w192) -> ()  [unwired: 1 out]
            n158 = event-data() -> ()  [unwired: 1 in, 5 out]
          }
          event "ADAM Scan Table": Mouse Down? {
            n159 = event-data() -> ()  [unwired: 5 out]
            n160 = Two Button Dialog(message="Are you sure that you want to Run the ADAM Scan table on this machine?", 1:"Run" ("F button name (\"Cancel\")"), 2:"Cancel" ("T button name (\"OK\")")) -> (T button?=w196:bool)
            n161 = case shown="False" w196 {
              frame False {
                n162 = global read "Constants_global.vi" "EnFlo SW Folder"() -> (w199:path)
                n163 = Build Path(base path=w199, name or relative path=path "ADAM Server/ADAM_scan_table.vi") -> (appended path=w202:path)
                n164 = Open VI Reference(vi path=w202) -> (vi reference=w204:refnum<vi>, error out=w201:errorcluster)  [unwired: 1 in, 4 out]
                n165 = property class="VI"(reference=w204, error in=w201, "Front Panel Window:Open"=TRUE) -> (reference out=w205:refnum<vi>, error out=w206:errorcluster)
                n166 = invoke class="VI" method="Run VI"(reference=w205, error in=w206, "Wait until done"=FALSE, "Auto Dispose Ref"=TRUE) -> (reference out=w207:refnum<vi>, error out=w208:errorcluster)  [unwired: 1 in, 3 out]
                n167 = Close Reference(reference=w207, error in (no error)=w208) -> ()  [unwired: 1 out]
              }
              frame True {
              }
            }
            n168 = event-data() -> ()  [unwired: 1 in, 2 out]
          }
          event "RW Trav Setup": Mouse Down? {
            n169 = event-data() -> ()  [unwired: 5 out]
            n170 = global read "Constants_global.vi" "EnFlo SW Folder"() -> (w213:path)
            n171 = Build Path(base path=w213, name or relative path=path "ADAM Serial/Instrument drivers/Traverses/~subVIs/Read_Write_Trav_Config.vi") -> (appended path=w214:path)
            n172 = Build Path(base path=w213, name or relative path=path "ADAM Serial/Instrument drivers/Traverses/~subVIs/DriveConfigGlobal.vi") -> (appended path=w215:path)
            n173 = flat-sequence {
              tunnel: w215 -> [w216]
              tunnel: w214 -> [w218]
              frame #0 {
                n174 = call "Open_Close_Front_Panel.ph.vi"("Front Panel Window:Open"=TRUE, "VI path"=w216) -> ()  [unwired: 2 out]
              }
              frame #1 {
                n175 = call "Open_Close_Front_Panel.ph.vi"("Front Panel Window:Open"=TRUE, "VI path"=w218) -> ()  [unwired: 2 out]
              }
            }
            n176 = event-data() -> ()  [unwired: 1 in, 5 out]
          }
          event "Hot Wire Calc": Mouse Down? {
            n177 = event-data() -> ()  [unwired: 5 out]
            n178 = global read "Constants_global.vi" "EnFlo SW Folder"() -> (w220:path)
            n179 = Build Path(base path=w220, name or relative path=path "Anemometry/Utilities/Hot_wire_Calculator.vi") -> (appended path=w223:path)
            n180 = call "Open_Close_Front_Panel.ph.vi"("Front Panel Window:Open"=TRUE, "VI path"=w223) -> ()  [unwired: 2 out]
            n181 = event-data() -> ()  [unwired: 1 in, 5 out]
          }
          event "Show Manual Sync": Mouse Down {
            w226 = path "Anemometry/Utilities/EnFlo_Data_Sync_Manual.vi"  # Anemometry\Utilities\EnFlo_Data_Sync_Manual.vi
            n182 = event-data() -> ()  [unwired: 9 out]
            n183 = global read "Constants_global.vi" "EnFlo SW Folder"() -> (w224:path)
            n184 = Build Path(base path=w224, name or relative path=w226) -> (appended path=w227:path)
            n185 = call "Open_Close_Front_Panel.ph.vi"("Front Panel Window:Open"=TRUE, "VI path"=w227) -> ()  [unwired: 2 out]
          }
          event "Hydrosonic Control": Mouse Down? {
            n186 = event-data() -> ()  [unwired: 5 out]
            n187 = global read "Constants_global.vi" "EnFlo SW Folder"() -> (w228:path)
            n188 = Build Path(base path=w228, name or relative path=path "Anemometry/Utilities/Hydrosonic_Manual.vi") -> (appended path=w231:path)
            n189 = call "Open_Close_Front_Panel.ph.vi"("Front Panel Window:Open"=TRUE, "VI path"=w231) -> ()  [unwired: 2 out]
            n190 = event-data() -> ()  [unwired: 1 in, 5 out]
          }
          event "Top Level Traverse": Mouse Down {
            w234 = path "Anemometry/Utilities/Top_Level_Move_Traverse.vi"  # Anemometry\Utilities\Top_Level_Move_Traverse.vi
            n191 = event-data() -> ()  [unwired: 9 out]
            n192 = global read "Constants_global.vi" "EnFlo SW Folder"() -> (w232:path)
            n193 = Build Path(base path=w232, name or relative path=w234) -> (appended path=w235:path)
            n194 = call "Open_Close_Front_Panel.ph.vi"("Front Panel Window:Open"=TRUE, "VI path"=w235) -> ()  [unwired: 2 out]
          }
          event "Post_Pro_Results_Hierarchy": Mouse Down {
            w238 = path "Anemometry/Utilities/Post_Pro_Results_Hierarchy.vi"  # Anemometry\Utilities\Post_Pro_Results_Hierarchy.vi
            n195 = event-data() -> ()  [unwired: 9 out]
            n196 = global read "Constants_global.vi" "EnFlo SW Folder"() -> (w236:path)
            n197 = Build Path(base path=w236, name or relative path=w238) -> (appended path=w239:path)
            n198 = call "Open_Close_Front_Panel.ph.vi"("Front Panel Window:Open"=TRUE, "VI path"=w239) -> ()  [unwired: 2 out]
          }
          event "Fast FID Valve": Mouse Down? {
            n199 = event-data() -> ()  [unwired: 5 out]
            n200 = global read "Constants_global.vi" "EnFlo SW Folder"() -> (w240:path)
            n201 = Build Path(base path=w240, name or relative path=path "ADAM Client/ADAM client VIs/Fast_FID_Valve_Control.vi") -> (appended path=w243:path)
            n202 = call "Open_Close_Front_Panel.ph.vi"("Front Panel Window:Open"=TRUE, "VI path"=w243) -> ()  [unwired: 2 out]
            n203 = event-data() -> ()  [unwired: 1 in, 5 out]
          }
          event "Preference Panel": Mouse Down? {
            n204 = event-data() -> ()  [unwired: 5 out]
            n205 = global read "Constants_global.vi" "EnFlo SW Folder"() -> (w244:path)
            n206 = Build Path(base path=w244, name or relative path=path "Anemometry/Utilities/Preference_Panel.vi") -> (appended path=w253:path)
            n207 = Open VI Reference(type specifier VI Refnum (for type only)=refnum<vi> refnum, vi path=w253) -> (vi reference=w246:refnum<vi>, error out=w247:errorcluster)  [unwired: 1 in, 3 out]
            n208 = property class="VI Interface Type 2"(reference=w246, error in=w247, "Front Panel Window:Open"=TRUE) -> (reference out=w249:refnum<vi>, error out=w250:errorcluster)
            n209 = call-by-ref "?"(reference=w249, error in=w250, "Mode"=Preference_Mode."Load, Edit then Save") -> (reference out=w251:refnum<vi>, error out=w252:errorcluster)
            n210 = Close Reference(reference=w251, error in (no error)=w252) -> ()  [unwired: 1 out]
            n211 = event-data("Discard?"=TRUE) -> ()  [unwired: 1 in, 4 out]
          }
          event "Gas Release Setup": Mouse Down? {
            n212 = event-data() -> ()  [unwired: 5 out]
            n213 = global read "Constants_global.vi" "EnFlo SW Folder"() -> (w260:path)
            n214 = Build Path(base path=w260, name or relative path=path "ADAM Client/Sub VIs/Gas_Setup.vi") -> (appended path=w267:path)
            n215 = Open VI Reference(type specifier VI Refnum (for type only)=refnum<vi> refnum, vi path=w267) -> (vi reference=w263:refnum<vi>, error out=w264:errorcluster)  [unwired: 1 in, 3 out]
            n216 = property class="VI Interface Type 3"(reference=w263, error in=w264, "Front Panel Window:Open"=TRUE) -> (reference out=w268:refnum<vi>, error out=w266:errorcluster)
            n217 = call-by-ref "?"(reference=w268, error in=w266) -> (reference out=w258:refnum<vi>, error out=w257:errorcluster)  [unwired: 9 in]
            n218 = Close Reference(reference=w258, error in (no error)=w257) -> ()  [unwired: 1 out]
            n219 = event-data("Discard?"=TRUE) -> ()  [unwired: 1 in, 4 out]
          }
          event "User Metadata": Mouse Down? {
            n220 = event-data() -> ()  [unwired: 5 out]
            n221 = global read "Constants_global.vi" "EnFlo SW Folder"() -> (w272:path)
            n222 = Build Path(base path=w272, name or relative path=path "ADAM Client/Sub VIs/User_Metadata.vi") -> (appended path=w279:path)
            n223 = Open VI Reference(type specifier VI Refnum (for type only)=refnum<vi> refnum, vi path=w279) -> (vi reference=w275:refnum<vi>, error out=w276:errorcluster)  [unwired: 1 in, 3 out]
            n224 = property class="VI Interface Type 3"(reference=w275, error in=w276, "Front Panel Window:Open"=TRUE) -> (reference out=w280:refnum<vi>, error out=w278:errorcluster)
            n225 = call-by-ref "?"(reference=w280, error in=w278) -> (reference out=w270:refnum<vi>, error out=w269:errorcluster)  [unwired: 9 in]
            n226 = Close Reference(reference=w270, error in (no error)=w269) -> ()  [unwired: 1 out]
            n227 = event-data("Discard?"=TRUE) -> ()  [unwired: 1 in, 4 out]
          }
          event "EnFlo Tunnel Setup": Mouse Down? {
            n228 = event-data() -> ()  [unwired: 5 out]
            n229 = global read "Constants_global.vi" "EnFlo SW Folder"() -> (w286:path)
            n230 = Build Path(base path=w286, name or relative path=path "ADAM Client/Sub VIs/EnFlo_Tunnel_Setup.vi") -> (appended path=w289:path)
            n231 = Open VI Reference(type specifier VI Refnum (for type only)=refnum<vi> refnum, vi path=w289) -> (vi reference=w283:refnum<vi>, error out=w282:errorcluster)  [unwired: 1 in, 3 out]
            n232 = call-by-ref "?"(reference=w283, error in=w282) -> (reference out=w285:refnum<vi>, error out=w284:errorcluster)  [unwired: 9 in]
            n233 = Close Reference(reference=w285, error in (no error)=w284) -> ()  [unwired: 1 out]
            n234 = event-data("Discard?"=TRUE) -> ()  [unwired: 1 in, 4 out]
          }
          event "Traverse Space": Mouse Down? {
            w300 = TRUE  # Show Panel?
            n235 = event-data() -> ()  [unwired: 5 out]
            n236 = global read "Constants_global.vi" "EnFlo SW Folder"() -> (w295:path)
            n237 = Build Path(base path=w295, name or relative path=path "Anemometry/Anemometry Sub Vis/Gen Trav/Traverse_Space.vi") -> (appended path=w298:path)
            n238 = global read "Trav_pos_global.vi" "Default Traverse Setup"() -> (w290:string)
            n239 = Open VI Reference(type specifier VI Refnum (for type only)=refnum<vi> refnum, vi path=w298) -> (vi reference=w299:refnum<vi>, error out=w291:errorcluster)  [unwired: 1 in, 3 out]
            n240 = call-by-ref "?"(reference=w299, error in=w291, "Show Panel?"=w300, "Traverse Setup"=w290) -> (reference out=w293:refnum<vi>, error out=w292:errorcluster)  [unwired: 8 in, 1 out]
            n241 = Close Reference(reference=w293, error in (no error)=w292) -> ()  [unwired: 1 out]
            n242 = event-data("Discard?"=TRUE) -> ()  [unwired: 1 in, 4 out]
          }
          event "EnFlo Arm": Mouse Down? {
            n243 = event-data() -> ()  [unwired: 5 out]
            n244 = global read "Constants_global.vi" "EnFlo SW Folder"() -> (w302:path)
            n245 = Build Path(base path=w302, name or relative path=path "Anemometry/Anemometry Sub Vis/Traverse vi's/EnFlo Tunnel specific/Check_EnFlo_Arm.vi") -> (appended path=w304:path)
            n246 = call "Open_Close_Front_Panel.ph.vi"("Front Panel Window:Open"=TRUE, "VI path"=w304) -> ()  [unwired: 2 out]
            n247 = event-data() -> ()  [unwired: 1 in, 2 out]
          }
          event "Trav 3D Move": Mouse Down? {
            n248 = event-data() -> ()  [unwired: 5 out]
            n249 = global read "Constants_global.vi" "EnFlo SW Folder"() -> (w312:path)
            n250 = Build Path(base path=w312, name or relative path=path "Anemometry/Anemometry Sub Vis/Gen Trav/3D_Traverse_move.vi") -> (appended path=w309:path)
            n251 = Strip Path(path=w309) -> (name=w308:string)  [unwired: 1 out]
            n252 = Open VI Reference(vi path=w308) -> (vi reference=w310:refnum<vi>, error out=w311:errorcluster)  [unwired: 1 in, 4 out]
            n253 = property class="VI"(reference=w310, error in=w311) -> (reference out=w306:refnum<vi>, error out=w305:errorcluster, "Front Panel Window:Open"=w307:bool)
            n254 = case shown="False" w307 {
              tunnel: w309 -> [w314 _]
              tunnel: w306 -> [_ w331]
              tunnel: w305 -> [_ w330]
              frame False {
                n255 = global read "Trav_pos_global.vi" "Work in Tunnel Coordinates?"() -> (w324:T47)
                n256 = global read "Trav_pos_global.vi" "Default Traverse Setup"() -> (w322:string)
                n257 = Open VI Reference(type specifier VI Refnum (for type only)=refnum<vi> refnum, vi path=w314) -> (vi reference=w318:refnum<vi>, error out=w319:errorcluster)  [unwired: 1 in, 3 out]
                n258 = property class="VI Interface Type 4"(reference=w318, error in=w319, "Front Panel Window:Open"=TRUE) -> (reference out=w315:refnum<vi>, error out=w316:errorcluster)
                n259 = call-by-ref "?"(reference=w315, error in=w316, "Mode"=Trav_mode."Read traverse position", "Work in Tunnel Coordinates"=w324, "Simulate/Run"=User_Specific_mode."Run VI", "Traverse name"=w322) -> (reference out=w320:refnum<vi>, error out=w321:errorcluster)  [unwired: 9 in, 3 out]
                n260 = Close Reference(reference=w320, error in (no error)=w321) -> ()  [unwired: 1 out]
              }
              frame True {
                n261 = property class="VI"(reference=w331, error in=w330, "Front Panel Window:Open"=TRUE) -> (reference out=w329:refnum<vi>, error out=w328:errorcluster)
                n262 = Close Reference(reference=w329, error in (no error)=w328) -> ()  [unwired: 1 out]
              }
            }
            n263 = event-data() -> ()  [unwired: 1 in, 5 out]
          }
          event "Multi Run Prog": Mouse Down? {
            n264 = event-data() -> ()  [unwired: 5 out]
            n265 = Open VI Reference(vi path="Multi_Run_Prog.vi") -> (vi reference=w337:refnum<vi>, error out=w336:errorcluster)  [unwired: 1 in, 4 out]
            n266 = property class="VI"(reference=w337, error in=w336, "Front Panel Window:Open"=TRUE) -> (reference out=w334:refnum<vi>, error out=w335:errorcluster)
            n267 = Close Reference(reference=w334, error in (no error)=w335) -> (error out=w332:errorcluster)
            n268 = Unbundle By Name(w332) -> ("status"=w339:bool)
            n269 = case shown="True" w339 {
              frame False {
              }
              frame True {
                n270 = global read "Constants_global.vi" "EnFlo SW Folder"() -> (w347:path)
                n271 = call "Setup_Filepath.vi"("Setup File Type"=Setup_Filetype."General", "Filename in"="Multi_Run_Filename.txt" ("name or relative path")) -> ("Filename Out"=w340:path)  [unwired: 1 out]
                n272 = Build Path(base path=w347, name or relative path=path "Anemometry/Multi_Run_Prog.vi") -> (appended path=w346:path)
                n273 = call "Read_File_Simple.vi"("Filename"=w340) -> ("string"=w345:string)  [unwired: 2 in, 7 out]
                n274 = String To Path(string=w345) -> (path=w343:path)
                n275 = call "Does_file_exist_(simple).vi"("Pathname"=w343) -> ("exists?"=w344:bool)
                n276 = case shown="False" w344 {
                  tunnel: w346 -> [w349 w361]
                  tunnel: w343 -> [_ w358]
                  frame False {
                    n277 = call "Open_Close_Front_Panel.ph.vi"("Front Panel Window:Open"=TRUE, "VI path"=w349) -> ()  [unwired: 2 out]
                  }
                  frame True {
                    n278 = Open VI Reference(type specifier VI Refnum (for type only)=refnum<vi> refnum, vi path=w361) -> (vi reference=w357:refnum<vi>, error out=w356:errorcluster)  [unwired: 1 in, 3 out]
                    n279 = property class="VI Interface Type 5"(reference=w357, error in=w356, "Front Panel Window:Open"=TRUE) -> (reference out=w354:refnum<vi>, error out=w355:errorcluster)
                    n280 = call-by-ref "?"(reference=w354, error in=w355, "Command filename"=w358, "Setup mode"=T45."Load Command File") -> (reference out=w353:refnum<vi>, error out=w352:errorcluster)  [unwired: 18 in]
                    n281 = Close Reference(reference=w353, error in (no error)=w352) -> ()  [unwired: 1 out]
                  }
                }
              }
            }
            n282 = event-data() -> ()  [unwired: 1 in, 5 out]
          }
          event "Calibration Prog": Mouse Down? {
            w363 = "Calibration.vi" ("name or relative path")
            n283 = event-data() -> ()  [unwired: 5 out]
            n284 = global read "Constants_global.vi" "EnFlo SW Folder"() -> (w369:path)
            n285 = Open VI Reference(vi path=w363) -> (vi reference=w367:refnum<vi>, error out=w366:errorcluster)  [unwired: 1 in, 4 out]
            n286 = Build Path(base path=w369, name or relative path="Anemometry") -> (appended path=w372:path)
            n287 = property class="VI"(reference=w367, error in=w366, "Front Panel Window:Open"=TRUE) -> (reference out=w364:refnum<vi>, error out=w365:errorcluster)
            n288 = Build Path(base path=w372, name or relative path=w363) -> (appended path=w370:path)
            n289 = Close Reference(reference=w364, error in (no error)=w365) -> (error out=w362:errorcluster)
            n290 = Unbundle By Name(w362) -> ("status"=w371:bool)
            n291 = case shown="True" w371 {
              tunnel: w370 -> [_ w374]
              tunnel: w362 -> [_ _]
              frame False {
              }
              frame True {
                n292 = stacked-sequence {
                  seq-local: [w380 _] -> [_ w387]
                  tunnel: w374 -> [_ w388]
                  frame #0 {
                    n293 = call "Setup_Filepath.vi"("Setup File Type"=Setup_Filetype."Calibration Setups", "Filename in"="Current_Setup.xls") -> ("Filename Out"=w375:path)  [unwired: 1 out]
                    n294 = call "Read_File_Simple.vi"("Filename"=w375) -> ("string"=w384:string)  [unwired: 2 in, 7 out]
                    n295 = Format Into String(format string="Calibration Setup File   %s", w375) -> (resulting string=w378:string)  [unwired: 2 in, 1 out]
                    n296 = call "Get_string_subset.vi"("String Name"=w378, "String to split"=w384, "File Label"="Raw data header") -> ("Output string"=w382:string)  [unwired: 1 in, 1 out]
                    n297 = call "Get_Characters_from_string.vi"("Input string"=w382, "Variable name"="Calib filename") -> ("Value"=w381:string)  [unwired: 1 in, 1 out]
                    n298 = call "String_to_Pathname.vi"("Input String"=w381) -> ("path"=w380:path)
                  }
                  frame #1 {
                    n299 = call "Does_file_exist_(simple).vi"("Pathname"=w387) -> ("exists?"=w386:bool)
                    n300 = case shown="True" w386 {
                      tunnel: w388 -> [w389 w404]
                      tunnel: w387 -> [_ w398]
                      frame False {
                        n301 = call "Open_Close_Front_Panel.ph.vi"("Front Panel Window:Open"=TRUE, "VI path"=w389) -> ()  [unwired: 2 out]
                      }
                      frame True {
                        w396 = TRUE ("Front Panel Window:Open")
                        n302 = Open VI Reference(type specifier VI Refnum (for type only)=refnum<vi> refnum, vi path=w404) -> (vi reference=w402:refnum<vi>, error out=w397:errorcluster)  [unwired: 1 in, 3 out]
                        n303 = property class="VI Interface Type 6"(reference=w402, error in=w397, "Front Panel Window:Open"=w396, "Front Panel Window:Auto Center (Deprecated)"=w396) -> (reference out=w401:refnum<vi>, error out=w400:errorcluster)
                        n304 = call-by-ref "?"(reference=w401, error in=w400, "Mode"=Calib_mode."Setup Front Panel", "Calib file"=w398) -> (reference out=w394:refnum<vi>, error out=w393:errorcluster)  [unwired: 15 in, 3 out]
                        n305 = property class="VI Interface Type 6"(reference=w394, error in=w393, "Front Panel Window:Auto Center (Deprecated)"=FALSE ("Front Panel Window:Auto Center")) -> (reference out=w392:refnum<vi>, error out=w391:errorcluster)
                        n306 = Close Reference(reference=w392, error in (no error)=w391) -> ()  [unwired: 1 out]
                      }
                    }
                  }
                }
              }
            }
            n307 = event-data() -> ()  [unwired: 1 in, 5 out]
          }
          event "stop": Mouse Down? {
            n308 = event-data() -> ()  [unwired: 5 out]
            n309 = flat-sequence {
              frame #0 {
                n310 = global write "Dynamic_call_global.ph.vi" "EnFlo Hub running?"(FALSE ("EnFlo Hub running?")) -> ()
              }
              frame #1 {
                n311 = Stop(stop? (T)=TRUE) -> ()
              }
            }
            n312 = event-data() -> ()  [unwired: 1 in, 4 out]
          }
          event "Rig_Control": Value Change {
            n313 = event-data() -> ("OldVal"=w408:cluster{"Ch Name":string, "Boolean":bool}[], "NewVal"=w407:cluster{"Ch Name":string, "Boolean":bool}[])  [unwired: 5 out]
            n314 = for {
              tunnel: w408 -> [w414] mode=indexing
              tunnel: w407 -> [w413] mode=indexing
              n315 = Unbundle By Name(w414) -> ("Ch Name"=w411:string, "Boolean"=w412:bool)
              n316 = Unbundle By Name(w413) -> ("Boolean"=w410:bool)  [unwired: 1 out]
              n317 = Not Equal?(x=w412, y=w410) -> (x != y?=w409:bool)
              n318 = case shown="True" w409 {
                tunnel: w411 -> [_ w416]
                tunnel: w410 -> [_ w423]
                frame False {
                }
                frame True {
                  n319 = Select(t="TRUE", s=w423, f="FALSE") -> (s? t:f=w415:string)
                  n320 = Select(t=1.0, s=w423, f=0.0) -> (s? t:f=w422:dbl)
                  n321 = Format Into String(format string="Are you sure you want to make %s %s?", w416, w415) -> (resulting string=w425:string)  [unwired: 2 in, 1 out]
                  n322 = Format Into String(format string="Make  %s  %s", w416, w415) -> (resulting string=w417:string)  [unwired: 2 in, 1 out]
                  n323 = Two Button Dialog(message=w425, 1:w417, 2:"Cancel" ("T button name (\"OK\")")) -> (T button?=w419:bool)
                  n324 = case shown="False" w419 {
                    tunnel: w416 -> [w430 _]
                    tunnel: w422 -> [w429 _]
                    frame False {
                      n325 = Build Array(w429) -> (w432:dbl[])
                      n326 = Build Array(w430) -> (w431:string[])
                      n327 = call "ASYNC_Adam_client.vi"("Values"=w432, "Channel Names"=w431) -> ()  [unwired: 2 out]
                    }
                    frame True {
                    }
                  }
                }
              }
            }
          }
          event Timeout {
            n328 = event-data() -> ()  [unwired: 4 out]
          }
        }
      }
    }
    "Numeric" <- w18
  }
  n329 = while {
    shift-left: _ -> [w438]
    shift-right: [w439] -> _
    shift-left: "Initialise" -> [w437]
    shift-right: [w440] -> _
    tunnel: "ADAM_Chs_to_Enable.txt" ("name or relative path") -> [w435]
    tunnel: "ADAM_Chs_to_View.txt" ("name or relative path") -> [w434]
    tunnel: w1 -> [w433]
    i -> [w436]
    stop <- TRUE continue-if-true
    n330 = case shown="\"Initialise\"" w437 {
      tunnel: ["End" "Initialise" "Wait for call remote sub vi occurrence" "Check type of VI to launch" w511 "Wait until remote sub vi is opened" "Update opened vis array" "Update opened vis array" "Update opened vis array" "Wait until remote sub vi is opened" "Wait for call remote sub vi occurrence"] -> w440
      tunnel: [w443 w455 w461 errorcluster {"status"=FALSE, "code"=0, "source"=""} ("error out") w507 w522 w552 w569 w584 w624 w644] -> w439
      tunnel: w438 -> [w443 w455 w461 _ w507 w522 _ _ _ w624 w644]
      tunnel: w437 -> [w445 _ _ _ _ _ _ _ _ _ _]
      tunnel: w436 -> [_ _ _ _ _ _ _ _ _ _ _]
      tunnel: w435 -> [_ _ w458 _ _ _ _ _ _ _ _]
      tunnel: w434 -> [_ _ w457 _ _ _ _ _ _ _ _]
      tunnel: w433 -> [w442 _ w456 _ _ _ _ _ _ _ _]
      frame "No match", Default {
        n331 = Current VI's Path() -> ()  [unwired: 1 out]
        n332 = Format Into String(format string="The Case\"%s\" was not Matched\nin VI named\n'%s\"" ("Format String"), w445, w442) -> (resulting string=w448:string)  [unwired: 2 in, 1 out]
        n333 = One Button Dialog(message=w448, button name ("OK")="STOP") -> (true=w446:bool)
        n334 = Stop(stop? (T)=w446) -> ()
      }
      frame "Never run" {
        # "These globals are here to make sure they stay in momory\nafter \"Preference Panel\" has finished running"
        n335 = call "Email_With_Log.vi"() -> ()  [unwired: 4 in, 3 out]
        n336 = call "Remember_value.vi"() -> ()  [unwired: 3 in, 1 out]
        n337 = call "Output_Trav_Pos.vi"() -> ()  [unwired: 5 in, 1 out]
        n338 = call "Read_Write_Local_table.vi"() -> ()  [unwired: 3 in, 3 out]
        n339 = call "Overhead_Factor.vi"() -> ()  [unwired: 4 in, 1 out]
        n340 = global read "Trav_pos_global.vi" "Dummy Measurement?"() -> (→"Dummy Measurement":bool)
        n341 = global read "PWAtasksGLOBAL.vi" "Analogue Dev Name"() -> (→"Analogue Dev Name":string)
        n342 = global read "Constants_global.vi" "All_Users"() -> (→"All Users":path)
        n343 = global read "Preference_global.vi" "Rig Setup"() -> (→"Rig Name":string)
      }
      frame "Initialise" {
        n344 = stacked-sequence {
          tunnel: w458 -> [_ _ _ _ w499]
          tunnel: w457 -> [_ _ _ _ w495]
          tunnel: w456 -> [w462 _ w484 _ _]
          frame #0 {
            n345 = Generate Occurrence() -> (w482:refnum<k4>)
            n346 = global write "Dynamic_call_global.ph.vi" "Call Remote Subvi"(w482) -> ()
            n347 = Generate Occurrence() -> (w481:refnum<k4>)
            n348 = global write "Dynamic_call_global.ph.vi" "Remote Subvi Opened"(w481) -> ()
            n349 = Initialize Array("", 0) -> (w479:string[])
            n350 = global write "Dynamic_call_global.ph.vi" "Opened VIs"(w479) -> ()
            n351 = global write "Email_transfer_global.vi" "Busy?"(FALSE ("Busy?")) -> ()
            n352 = Current VI's Path() -> ()  [unwired: 1 out]
            n353 = Strip Path(path=w462) -> (stripped path=w470:path)  [unwired: 1 out]
            n354 = Build Path(base path=w470, name or relative path="Utilities") -> (appended path=w468:path)
            n355 = Build Path(base path=w468, name or relative path="Preference_Panel.vi") -> (appended path=w467:path)
            n356 = Get Date/Time In Seconds() -> (seconds since 1Jan1904=w477:timestamp)
            n357 = To Double Precision Float(number=w477) -> (double precision float=w476:dbl)
            n358 = Open VI Reference(type specifier VI Refnum (for type only)=refnum<vi> refnum, vi path=w467) -> (vi reference=w472:refnum<vi>, error out=w473:errorcluster)  [unwired: 1 in, 3 out]
            n359 = global write "Meas_global.vi" "Start Time of experiment"(w476) -> ()
            n360 = global write "Meas_global.vi" "Post Process"(Post_Process."Post Process Raw Data File" ("Post Process")) -> ()
            n361 = call-by-ref "?"(reference=w472, error in=w473, "Mode"=Preference_Mode."Load Preferences from file") -> (reference out=w474:refnum<vi>, error out=w475:errorcluster)
            n362 = Close Reference(reference=w474, error in (no error)=w475) -> ()  [unwired: 1 out]
          }
          frame #1 {
            w483 = TRUE  # OK
            n363 = call "Get_users_email_addresses.vi"("OK"=w483) -> ()  [unwired: 5 out]
          }
          frame #2 {
            n364 = Current VI's Path() -> ()  [unwired: 1 out]
            n365 = Open VI Reference(vi path=w484) -> (vi reference=w492:refnum<vi>, error out=w491:errorcluster)  [unwired: 1 in, 4 out]
            n366 = call "Last_modified_date.vi"("Update Now"=TRUE) -> ("RevisionString"=w485:string)  [unwired: 1 out]
            n367 = property class="VI"(reference=w492, error in=w491, "Front Panel Window:Open"=TRUE, "Front Panel Window:Is Frontmost"=FALSE) -> (reference out=w490:refnum<vi>, error out=w489:errorcluster)
            n368 = global write "Meas_global.vi" "ProgRevisionInfo"(w485) -> ()
            n369 = Close Reference(reference=w490, error in (no error)=w489) -> ()  [unwired: 1 out]
          }
          frame #3 {
            n370 = global write "Dynamic_call_global.ph.vi" "EnFlo Hub running?"(TRUE ("EnFlo Hub running?")) -> ()
          }
          frame #4 {
            n371 = global read "Constants_global.vi" "All_Users"() -> (w496:path)
            n372 = Build Path(base path=w496, name or relative path=w495) -> (appended path=w498:path)
            n373 = Build Path(base path=w496, name or relative path=w499) -> (appended path=w501:path)
            n374 = call "Read_File_Simple.vi"("Filename"=w498) -> ("string"=w497:string)  [unwired: 2 in, 7 out]
            n375 = call "Read_File_Simple.vi"("Filename"=w501) -> ("string"=w502:string)  [unwired: 2 in, 7 out]
            n376 = call "Get_array_values_fr_String.vi"("String Value"=w497) -> ("String array"=→"List of ADAM channels to view":string[])  [unwired: 1 out]
            n377 = call "Get_array_values_fr_String.vi"("String Value"=w502) -> ("String array"=→"List of ADAM control channels":string[])  [unwired: 1 out]
          }
        }
        "Iterations" <- 0 ("Iterations")
      }
      frame "Wait for call remote sub vi occurrence" {
        n378 = global read "Dynamic_call_global.ph.vi" "Call Remote Subvi"() -> (w505:refnum<k4>)
        n379 = Wait on Occurrence(2:w505) -> ()  [unwired: 3 out]
      }
      frame "Check type of VI to launch" {
        n380 = global read "Dynamic_call_global.ph.vi" "VI name to launch"() -> (w509:string)
        n381 = Match Pattern(string=w509, regular expression=";") -> (before substring=w506:string, after substring=w508:string)  [unwired: 3 out]
        n382 = case shown="\"Other\", Default" w506 {
          tunnel: ["Open vi" "Open application reference" "Open Analogue input server" w519] -> w511
          tunnel: [w514 w516 w518 w520] -> w510
          tunnel: w509 -> [w514 _ _ _]
          tunnel: w508 -> [_ w516 w518 w520]
          tunnel: w506 -> [_ _ _ w519]
          frame "Other", Default {
          }
          frame "Open Application Reference" {
          }
          frame "Open Analogue Input VI" {
          }
          frame "Open LDA PWA & An" {
          }
        }
        "VI Name" <- w510
      }
      frame "Open application reference" {
        n383 = local read "VI Name"() -> (w523:string)
        n384 = Match Pattern(string=w523, regular expression=";") -> (before substring=w531:string, after substring=w532:string)  [unwired: 3 out]
        n385 = Decimal String To Number(string=w532) -> (number=w533:i32)  [unwired: 3 out]
        n386 = To Unsigned Long Integer(number=w533) -> (unsigned 32bit integer=w530:u32)
        n387 = call "App_Ref_Global.vi"("Mode"=App_Global."Read Global") -> ("Output Array"=w529:T49[])  [unwired: 1 in, 1 out]
        n388 = Open Application Reference(10:w530, 11:w531) -> (0:w524:errorcluster, 3:w528:refnum<vi>)  [unwired: 1 in, 1 out]
        n389 = for {
          tunnel: w529 -> [w535] mode=indexing
          tunnel: w523 -> [w539]
          tunnel: w528 -> [w537]
          tunnel: [w536] -> w527 mode=indexing
          n390 = Unbundle By Name(w535) -> ("Server IP & Port No"=w540:string)
          n391 = Equal?(x=w540, y=w539) -> (x = y?=w538:bool)
          n392 = case shown="False" w538 {
            tunnel: w537 -> [_ w544]
            tunnel: [w541 w543] -> w536
            tunnel: w535 -> [w541 w542]
            frame False {
            }
            frame True {
              n393 = Bundle By Name(cluster=w542, "Application reference"=w544) -> (w543:T49)
            }
          }
        }
        n394 = global write "Dynamic_call_global.ph.vi" "Error Cluster"(w524) -> ()
        n395 = call "App_Ref_Global.vi"("Input Array"=w527, "Mode"=App_Global."Write to Global") -> ()  [unwired: 2 out]
      }
      frame "Open Analogue input server" {
        n396 = local read "VI Name"() -> (w549:string)
        n397 = call "Get_link_info.vi"("VI Name"=w549) -> ("Path name"=w546:path, "Application reference"=w547:refnum<vi>, "Local Call?"=w548:bool)  [unwired: 1 out]
        n398 = global read "Dynamic_call_global.ph.vi" "Analogue Input"() -> (w551:refnum<vi>)
        n399 = case shown="True" w548 {
          tunnel: w551 -> [w557 w561]
          tunnel: [w553 w560] -> w550
          tunnel: [w556 w559] -> w552
          tunnel: w549 -> [w555 _]
          tunnel: w547 -> [w554 _]
          tunnel: w546 -> [_ w558]
          frame False {
            n400 = Open VI Reference(type specifier VI Refnum (for type only)=w557, application reference (local)=w554, vi path=w555) -> (vi reference=w553:refnum<vi>, error out=w556:errorcluster)  [unwired: 1 in, 2 out]
          }
          frame True {
            n401 = Open VI Reference(type specifier VI Refnum (for type only)=w561, vi path=w558) -> (vi reference=w560:refnum<vi>, error out=w559:errorcluster)  [unwired: 1 in, 3 out]
          }
        }
        n402 = global write "Dynamic_call_global.ph.vi" "Analogue Input"(w550) -> ()
      }
      frame "Open LDA PWA & An" {
        n403 = local read "VI Name"() -> (w566:string)
        n404 = call "Get_link_info.vi"("VI Name"=w566) -> ("Path name"=w563:path, "Application reference"=w564:refnum<vi>, "Local Call?"=w565:bool)  [unwired: 1 out]
        n405 = global read "Dynamic_call_global.ph.vi" "Take LDA PWA & An"() -> (w568:refnum<vi>)
        n406 = case shown="True" w565 {
          tunnel: w568 -> [w574 w578]
          tunnel: [w570 w577] -> w567
          tunnel: [w573 w576] -> w569
          tunnel: w566 -> [w572 _]
          tunnel: w564 -> [w571 _]
          tunnel: w563 -> [_ w575]
          frame False {
            n407 = Open VI Reference(type specifier VI Refnum (for type only)=w574, application reference (local)=w571, vi path=w572) -> (vi reference=w570:refnum<vi>, error out=w573:errorcluster)  [unwired: 1 in, 2 out]
          }
          frame True {
            n408 = Open VI Reference(type specifier VI Refnum (for type only)=w578, vi path=w575) -> (vi reference=w577:refnum<vi>, error out=w576:errorcluster)  [unwired: 1 in, 3 out]
          }
        }
        n409 = global write "Dynamic_call_global.ph.vi" "Take LDA PWA & An"(w567) -> ()
      }
      frame "Open vi" {
        n410 = local read "VI Name"() -> (w583:string)
        n411 = call "Get_link_info.vi"("VI Name"=w583) -> ("Path name"=w582:path, "Application reference"=w581:refnum<vi>, "Local Call?"=w580:bool)  [unwired: 1 out]
        n412 = case shown="\"GPIB_Server.vi\"" w583 {
          tunnel: [w585 w594 w606] -> w584
          tunnel: w583 -> [w590 w593 w610]
          tunnel: w582 -> [_ _ w607]
          tunnel: w581 -> [_ w592 w609]
          tunnel: w580 -> [_ w591 w608]
          frame "No Match", Default {
            n413 = Format Into String(format string="VI named \"%s\" Not matched" ("Format String"), w590) -> (resulting string=w587:string)  [unwired: 2 in, 1 out]
            n414 = Bundle By Name(cluster=errorcluster {"status"=FALSE, "code"=0, "source"=""} ("error out"), "source"=w587, "status"=TRUE ("Bundle Element")) -> (w585:errorcluster)
          }
          frame "Program_Active_server.vi" {
            n415 = global read "Dynamic_call_global.ph.vi" "Program Active server"() -> (w596:refnum<vi>)
            n416 = case shown="True" w591 {
              tunnel: w596 -> [w601 w605]
              tunnel: [w600 w604] -> w595
              tunnel: [w599 w603] -> w594
              tunnel: w593 -> [w598 w602]
              tunnel: w592 -> [w597 _]
              frame False {
                n417 = Open VI Reference(type specifier VI Refnum (for type only)=w601, application reference (local)=w597, vi path=w598) -> (vi reference=w600:refnum<vi>, error out=w599:errorcluster)  [unwired: 1 in, 2 out]
              }
              frame True {
                n418 = Open VI Reference(type specifier VI Refnum (for type only)=w605, vi path=w602) -> (vi reference=w604:refnum<vi>, error out=w603:errorcluster)  [unwired: 1 in, 3 out]
              }
            }
            n419 = global write "Dynamic_call_global.ph.vi" "Program Active server"(w595) -> ()
          }
          frame "GPIB_Server.vi" {
            n420 = global read "Dynamic_call_global.ph.vi" "GPIB_Server.vi"() -> (w612:refnum<vi>)
            n421 = case shown="False" w608 {
              tunnel: w612 -> [w617 w621]
              tunnel: [w616 w620] -> w611
              tunnel: [w615 w619] -> w606
              tunnel: w610 -> [w613 _]
              tunnel: w609 -> [w614 _]
              tunnel: w607 -> [_ w618]
              frame False {
                n422 = Open VI Reference(type specifier VI Refnum (for type only)=w617, application reference (local)=w614, vi path=w613) -> (vi reference=w616:refnum<vi>, error out=w615:errorcluster)  [unwired: 1 in, 2 out]
              }
              frame True {
                n423 = Open VI Reference(type specifier VI Refnum (for type only)=w621, vi path=w618) -> (vi reference=w620:refnum<vi>, error out=w619:errorcluster)  [unwired: 1 in, 3 out]
              }
            }
            n424 = global write "Dynamic_call_global.ph.vi" "GPIB_Server.vi"(w611) -> ()
          }
        }
      }
      frame "Update opened vis array" {
        w626 = TRUE  # Dialog Box
        n425 = local read "VI Name"() -> (w625:string)
        n426 = Unbundle By Name(w624) -> ("status"=w629:bool, "source"=w627:string)
        n427 = case shown="True" w629 {
          tunnel: w624 -> [w631 w640]
          tunnel: [w631 w639] -> w628
          tunnel: w625 -> [w632 w635]
          tunnel: w627 -> [_ w638]
          frame False {
            n428 = To Upper Case(1:w632) -> (0:w630:string)
            n429 = global read "Dynamic_call_global.ph.vi" "Opened VIs"() -> (w633:string[])
            n430 = Build Array (concatenate)(w633, w630) -> (w634:string[])
            n431 = global write "Dynamic_call_global.ph.vi" "Opened VIs"(w634) -> ()
          }
          frame True {
            n432 = Concatenate Strings(w635, " " ("Substring"), w638) -> (w636:string)
            n433 = Bundle By Name(cluster=w640, "source"=w636) -> (w639:errorcluster)
          }
        }
        n434 = call "EnFlo_Error_Handler.vi"("error in (no error)"=w628, "Error Type"="Dynamic Call", "Dialog Box (T)"=w626) -> ()  [unwired: 3 out]
      }
      frame "Wait until remote sub vi is opened" {
        n435 = global read "Dynamic_call_global.ph.vi" "Remote Subvi Opened"() -> (w645:refnum<k4>)
        n436 = local read "Iterations"() -> (w643:i32)
        n437 = Increment(x=w643) -> (x+1=w642:i32)
        n438 = local write "Iterations"(w642) -> ()
        n439 = Set Occurrence(w645) -> ()
      }
    }
  }
  n440 = while {
    tunnel: w1 -> [_]
    i -> [w646]
    stop <- FALSE stop-if-true
    n441 = stacked-sequence {
      tunnel: w646 -> [_ w698]
      frame #0 {
        n442 = global read "Dynamic_call_global.ph.vi" "EnFlo Hub running?"() -> (w650:bool)
        n443 = Equal?(x="Tab Control", y=T1."Adam Table" ("Tab Control")) -> (x = y?=w651:bool)
        n444 = And(x=w651, y=w650) -> (x .and. y?=w649:bool)
        n445 = case shown="True" w649 {
          frame True {
            n446 = local read "List of ADAM channels to view"() -> (w660:string[])
            n447 = local read "List of ADAM control channels"() -> (w663:string[])
            n448 = Build Array (concatenate)(w663, w660) -> (w662:string[])
            n449 = call "Get_Current_Scan_client.vi"("ADAM Ch Names"=w662) -> ("Ch Description Array"=w657:T51[], "Numerical Values"=w661:dbl[])  [unwired: 2 out]
            n450 = Array Size(array=w663) -> (size(s)=w658:i32)
            n451 = Array Subset(array=w657, index=w658) -> (w656:T51[])  [unwired: 1 in]
            n452 = Array Subset(array=w661, index=w658) -> (w655:dbl[])  [unwired: 1 in]
            n453 = for {
              tunnel: w656 -> [w670] mode=indexing
              tunnel: [w669] -> w654 mode=indexing
              tunnel: cluster{"Ch Name":string, "Numeric":dbl} {"Ch Name"="", "Numeric"=0.0} ("Cluster") -> [w668]
              tunnel: w655 -> [w666] mode=indexing
              n454 = Unbundle By Name(w670) -> ("Ch Name"=w667:string)
              n455 = Bundle By Name(cluster=w668, "Ch Name"=w667, "Numeric"=w666) -> (w669:cluster{"Ch Name":string, "Numeric":dbl})
            }
            "Current Values" <- w654
            n456 = for {
              N: w658 -> [_]
              tunnel: cluster{"Ch Name":string, "Boolean":bool} {"Ch Name"="", "Boolean"=FALSE} ("Cluster") -> [w677]
              tunnel: w657 -> [w676] mode=indexing
              tunnel: w661 -> [w674] mode=indexing
              tunnel: [w671] -> w664 mode=indexing
              n457 = Unbundle By Name(w676) -> ("Ch Name"=w675:string)
              n458 = Greater?(x=w674, y=0.5) -> (0:w672:bool)
              n459 = Bundle By Name(cluster=w677, "Ch Name"=w675, "Boolean"=w672) -> (w671:cluster{"Ch Name":string, "Boolean":bool})
            }
            n460 = local write "Rig_Control"(w664) -> ()
          }
          frame False {
          }
        }
      }
      frame #1 {
        w696 = 300 ("y")
        n461 = global read "Trav_pos_global.vi" "Top level setup filename"() -> (w681:path)
        n462 = Quotient & Remainder(x=w698, y=86400) -> (x-y*floor(x/y)=w699:i32)  [unwired: 1 out]
        n463 = Quotient & Remainder(x=w698, y=21600) -> (x-y*floor(x/y)=w695:i32)  [unwired: 1 out]
        n464 = Equal?(x=path "", y=w681) -> (x = y?=w680:bool)
        n465 = Equal?(x=w699, y=w696) -> (x = y?=w693:bool)
        n466 = Equal?(x=w696, y=w695) -> (x = y?=w694:bool)
        n467 = feedback-in #1(w680) -> ()
        n468 = feedback #1() -> (w679:bool)  [unwired: 1 in]
        n469 = Or(x=w693, y=w694) -> (x .or. y?=w686:bool)
        n470 = Compound Arithmetic op=AND(w680, invert w679) -> (w678:bool)
        n471 = Select(t=3 ("Months of History to backup"), s=w693, f=1) -> (s? t:f=w690:i32)
        n472 = global read "Preference_global.vi" "Server Comms"() -> (w688:T50)
        n473 = Equal?(x=w688, y=Server_Comms."Server Link Healthy" ("Server Comms")) -> (x = y?=w687:bool)
        n474 = And(x=w686, y=w687) -> (x .and. y?=w684:bool)
        n475 = Compound Arithmetic op=OR(w678, "Sync to server now", w684) -> (w683:bool)
        n476 = case shown="True" w683 {
          tunnel: w690 -> [_ w701]
          frame False {
          }
          frame True {
            n477 = stacked-sequence {
              tunnel: w701 -> [w704 _]
              frame #0 {
                w702 = TRUE  # Check Updates on Server?
                w703 = TRUE  # Get all Server Files
                n478 = call "Backup_Client.vi"("Check Updates on Server?"=w702, "Get all Server Files"=w703, "Months of History to backup"=w704) -> ()  [unwired: 1 out]
              }
              frame #1 {
                n479 = local write "Sync to server now"(FALSE ("Sync to server now")) -> ()
              }
            }
          }
        }
      }
    }
    n480 = Wait (ms)(milliseconds to wait=u32 1000) -> ()  [unwired: 1 out]
  }
